vi "Excitation.vi"() -> ()   [LabVIEW 2016]
uses:
  controls/EnumFGVHDT.ctl
  controls/Enum.ctl
  Course Project/support/Message Queue/Message Cluster.ctl
  <vilib>/rvi/errors/niLvFpgaAdjustHostInterfaceError.vi
  <vilib>/rvi/interface/common/niFpgaWaitOnOcc.vi
  <vilib>/RVI Host/nirviSupport.llb/nirviErrorClusterFromErrorCode.vi
  <vilib>/regexp/Match Regular Expression.xnode
  <vilib>/rvi/interface/nirviReadWriteControl/nirviReadWriteControl.xnode
  controls/FPGAVIreferenceTypeDef.ctl
  FPGA Bitfiles/qnmController797_usbRIO_controllerFPGAmu.lvbitx
  <vilib>/rvi/interface/nirviMethod/nirviMethod.xnode
  controls/FPGAVIreferenceTypeDefScanEngine.ctl
  Course Project/support/Message Queue/Message Queue.lvlib
  <vilib>/Analysis/NI_AAL_SigProc.lvlib
  <vilib>/rvi/errors/niLvFpgaMergeErrorWithErrorCode.vi
  NiFpgaLv.dll
  <vilib>/rvi/interface/nirviMethod/StockFPGA_InlinedMethodWaitForSingleIRQ.vi
  Course Project/support/User Event - Stop/User Event - Stop.lvlib
  <vilib>/FPGAPlugInAG/USB-7856R OEM/niLvFpga_AcknowledgeIrq_USB-7856R OEM.vi
  <vilib>/FPGAPlugInAG/USB-7856R OEM/niLvFpga_ConfigureFifo_USB-7856R OEM.vi
  <vilib>/FPGAPlugInAG/USB-7856R OEM/niLvFpga_StartFifo_USB-7856R OEM.vi
  <vilib>/FPGAPlugInAG/USB-7856R OEM/niLvFpga_ReadFifo_USB-7856R OEM.vi
  <vilib>/FPGAPlugInAG/USB-7856R OEM/niLvFpga_StopFifo_USB-7856R OEM.vi
  <vilib>/FPGAPlugInAG/USB-7856R OEM/niLvFpga_WaitOnIrq_USB-7856R OEM.vi
panel:
  in  "ort.bgc.p.waitTicks":u32=4096
  in  "heartBeatSimParams":T1={"curveParams"={"amplitude"=0.2, "peakHeight"=0.05, "cycleLength"=0, "snapIn"=0.001, "adhesion"=0.03, "peakShift"=0, "noiseAmplitude"=0.001, "asymmetry"=0.1}, "cantileverParams"={"samplingRate"=1000000.0, "cantileverFreq"=500000.0, "qFactor"=2.0}} {"cantileverParams"."cantileverFreq" format="%#_6p"; "cantileverParams"."samplingRate" format="%#_6p"}
  in  "lineFitThreshold":dbl=0.02
  in  "intOutMAEnable":bool=TRUE
  in  "Sensitivities":cluster{"Input":dbl, "Output":dbl}={"Input"=0.001506, "Output"=0.00030517578125} {"Output" format="%#_7p"}
  in  "ExcitationTab":enum32{"Page 1"}(tab)
  in  "Excitation enable?":bool caption="Enabling"
  in  "Background":bool
  in  "Signal":u16(ring) items=["Sine Wave", "Triangle Wave", "Square Wave", "Sawtooth Wave", "Heartbeat Signal"]
  in  "Synchronization":T2={"Lower"=0, "Upper"=10000, "Use SyncPoint"=FALSE, "syncPoint"=1000, "Average Band"=4} {"Average Band" items=["1", "2", "4", "16", "32", "64", "128", "256"]}
  out "Graph":dbl[](graph)
  in  "Excitation":T3={"Frequency"=1000.0, "Amplitude"=1e-07, "DC Offset"=0.0, "Cut Off"=40.0, "RaPF"=FALSE, "Shift"=0.0} {"Shift" min=-100.0 max=100.0 format="%_1p%"; "Cut Off" format="%.0p%"; "DC Offset" min=0.0 max=10.0 format="%_3pV"; "Amplitude" min=-10.0 max=10.0 format="%_3pV"; "Frequency" min=0.0 max=100000000.0 format="%.1pHz"}
  in  "Background-":cluster{"Lift Height":dbl, "Average Count":u16}={"Lift Height"=3e-08, "Average Count"=12} {"Average Count" items=["1", "2", "4", "8", "16", "32", "64", "128", "256", "512", "1024", "2048", "4096", "8192", "16384"]; "Lift Height" format="%_3pm"}
  in  "Type":u16(ring) items=["ZPiezo", "Photothermal"]
  in  "Display":u16(ring) items=["Excitation", "Background"]
  in  "Request":enum16{"Never", "End of line", "End of frame"}(ring)
  in  "Correction":bool=TRUE
  # "Excitation"
  # "Background"
  # "Background/Scan"
  # "Maximum search"
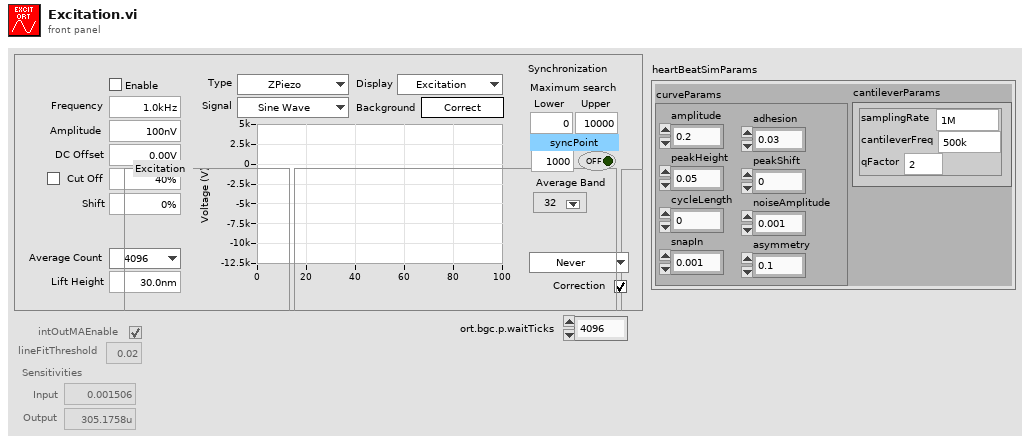
[diagram p1: front panel]
types:
  T1 = cluster{"curveParams":cluster{"amplitude":dbl, "peakHeight":dbl, "cycleLength":u16, "snapIn":dbl, "adhesion":dbl, "peakShift":u16, "noiseAmplitude":dbl, "asymmetry":dbl}, "cantileverParams":cluster{"samplingRate":dbl, "cantileverFreq":dbl, "qFactor":dbl}}
  T2 = cluster{"Lower":u16, "Upper":u16, "Use SyncPoint":bool, "syncPoint":u16, "Average Band":u16}
  T3 = cluster{"Frequency":dbl, "Amplitude":dbl, "DC Offset":dbl, "Cut Off":dbl, "RaPF":bool, "Shift":dbl}
  T4 = typedef "EnumFGVHDT.ctl" = enum16{"Init", "Read", "Write", "Push", "Pop"}
  T5 = typedef "Message Queue.lvlib/All Message Queues.ctl" = cluster{"IU":refnum<queue>}
  T6 = cluster{"Initialization":bool, "Ctrl":refnum<vi>}
  T7 = typedef "Enum.ctl" = enum16{"Init", "Read", "Write"}
  T8 = typedef "Message Queue.lvlib/Message Cluster.ctl" = cluster{"Message":string, "Données de message":variant}
  T9 = cluster{"upperLimit":fxp<+/-,28,4>, "lowerLimit":fxp<+/-,28,4>}
  T10 = enum8{"Enabled", "Disabled", "Disabled and Grayed Out"}
  T11 = cluster{"maxSearchLower":u16, "maxSearchUpper":u16}
  T12 = enum32{"Bad", "Idle", "Run top level", "Running"}
  T13 = cluster{"DC Offset":dbl, "amplitude":dbl, "frequency":dbl, "Signal Type":u16, "cutoff":dbl, "RaPF":bool, "shift":dbl}
  T14 = cluster{"Excitation":cluster{"Frequency":dbl, "Amplitude":dbl, "DC Offset":dbl, "Cut Off":dbl, "RaPF":bool, "Shift":dbl}, "Background":cluster{"Lift Height":dbl, "Average Count":u16}, "Signal":u16}
  T15 = cluster{"DC Offset":dbl, "amplitude":dbl, "frequency":dbl, "Signal Type":u16, "cutoff":dbl, "RaPF":bool}
  T16 = typedef "FPGAVIreferenceTypeDef.ctl" = refnum<k20>
  T17 = cluster{"hdt.int.s.transferSource":u8, "hdt.int.p.useInternalMemStartPos":bool, "hdt.int.p.memStartPos":fxp<+,14,14>, "hdt.int.p.readLength":u16, "hdt.int.p.readFwd":bool, "hdt.int.p.memReadDec":u16, "hdt.int.p.startTransfer":bool}
  T18 = cluster{"ort.p.winSizeP2":u16, "ort.p.syncPoint":u16, "ort.p.useSyncPoint":bool, "ort.p.bypassAvg":bool, "ort.p.searchBounds":cluster{"maxSearchLower":u16, "maxSearchUpper":u16}}
  T19 = typedef "FPGAVIreferenceTypeDefScanEngine.ctl" = refnum<k20>
  T20 = cluster{"calibName":string[], "calibParameters":cluster{"Sensitivity":cluster{"Sens X":dbl, "Sens Y":dbl, "Sens Z":dbl}, "Range":cluster{"Range X":dbl, "Range Y":dbl, "Range Z":dbl}, "HV gain":cluster{"HV gain X":dbl, "HV gain Y":dbl, "HV gain Z":dbl}}[], "calibIndex":i32}
  T21 = cluster{"Sensitivity":cluster{"Sens X":dbl, "Sens Y":dbl, "Sens Z":dbl}, "Range":cluster{"Range X":dbl, "Range Y":dbl, "Range Z":dbl}, "HV gain":cluster{"HV gain X":dbl, "HV gain Y":dbl, "HV gain Z":dbl}}[]
  T22 = cluster{"Sensitivity":cluster{"Sens X":dbl, "Sens Y":dbl, "Sens Z":dbl}, "Range":cluster{"Range X":dbl, "Range Y":dbl, "Range Z":dbl}, "HV gain":cluster{"HV gain X":dbl, "HV gain Y":dbl, "HV gain Z":dbl}}
  T23 = cluster{"liftHeight":fxp<+/-,15,4>, "disengagePos":fxp<+/-,22,1>}
  T24 = cluster{"maxSearchLower":u16, "maxSearchUpper":u16, "useSyncPoint":bool, "syncPoint":u16, "syncAverageBand":u16}
  T25 = cluster{"inputSensitivity":dbl, "outputSensitivity":dbl}
  T26 = cluster{"intOutMAEnable":bool, "bgcAverageCount":u16, "waveSize":u32, "resetBGC":bool, "liftHeight":fxp<+/-,15,4>}
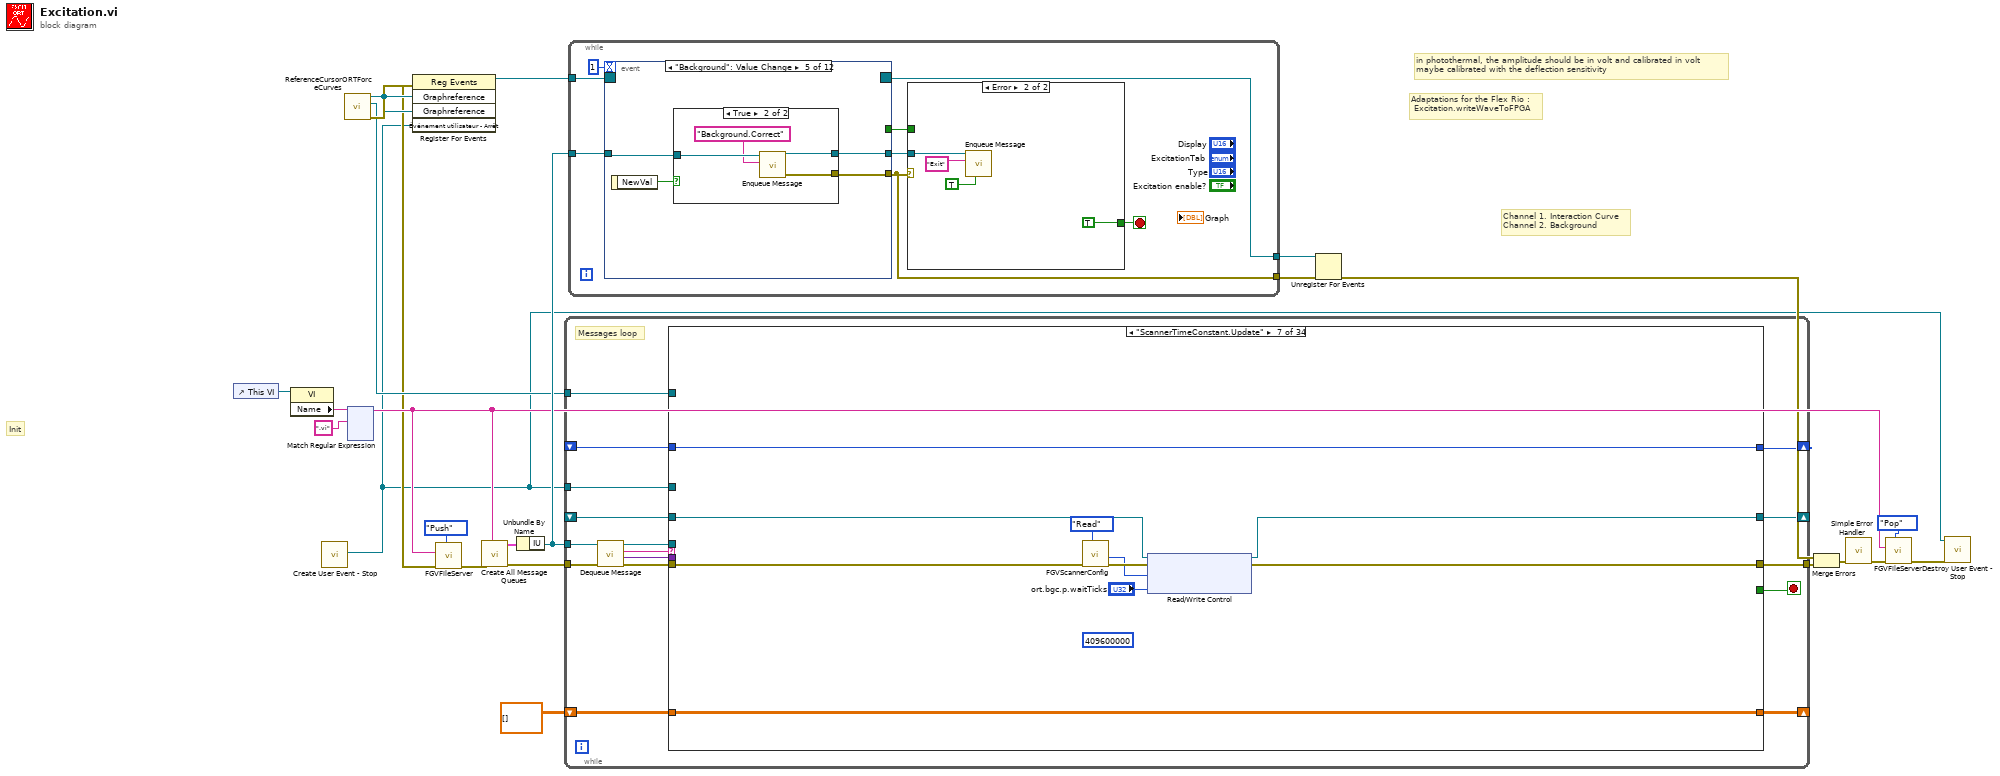
[diagram p0: block diagram]
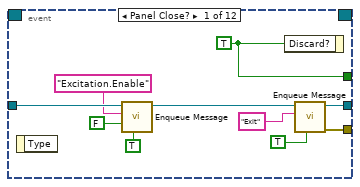
[diagram p3: hidden frame]
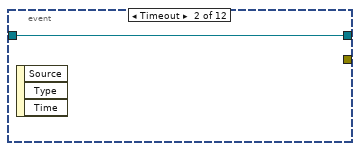
[diagram p4: hidden frame]
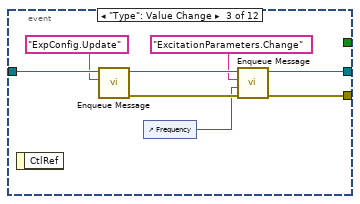
[diagram p5: hidden frame]
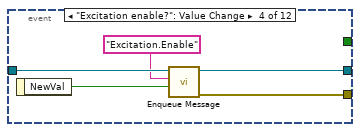
[diagram p6: hidden frame]
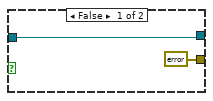
[diagram p7: hidden frame]
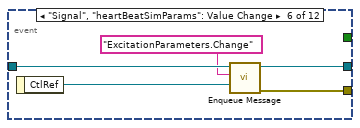
[diagram p8: hidden frame]
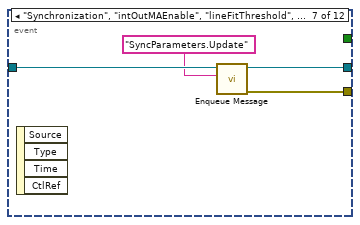
[diagram p9: hidden frame]
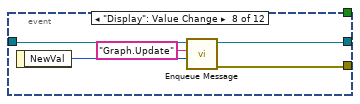
[diagram p10: hidden frame]
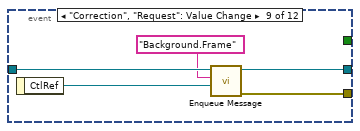
[diagram p11: hidden frame]
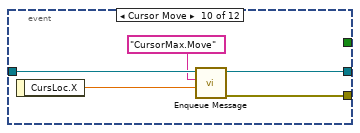
[diagram p12: hidden frame]
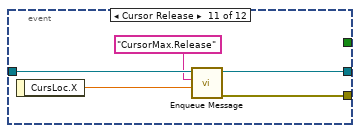
[diagram p13: hidden frame]
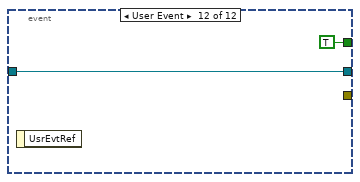
[diagram p14: hidden frame]
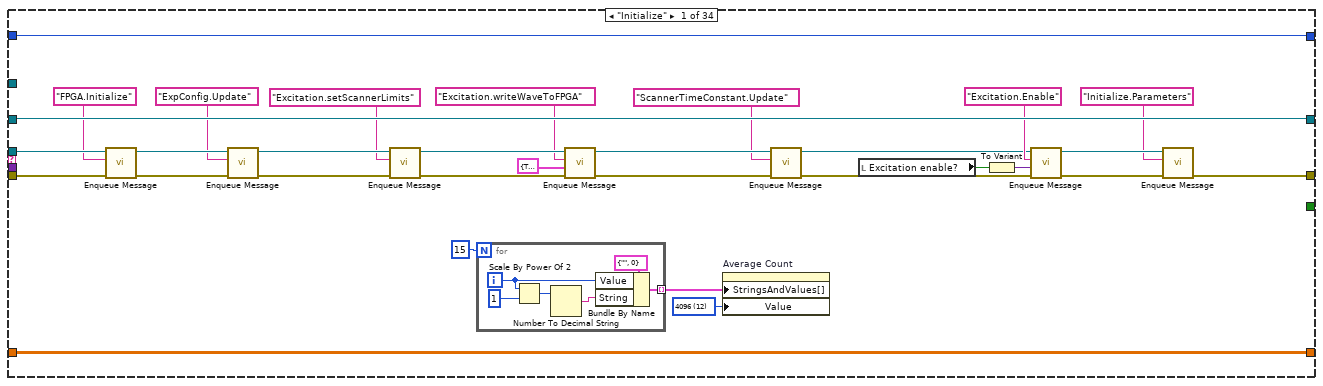
[diagram p15: hidden frame]
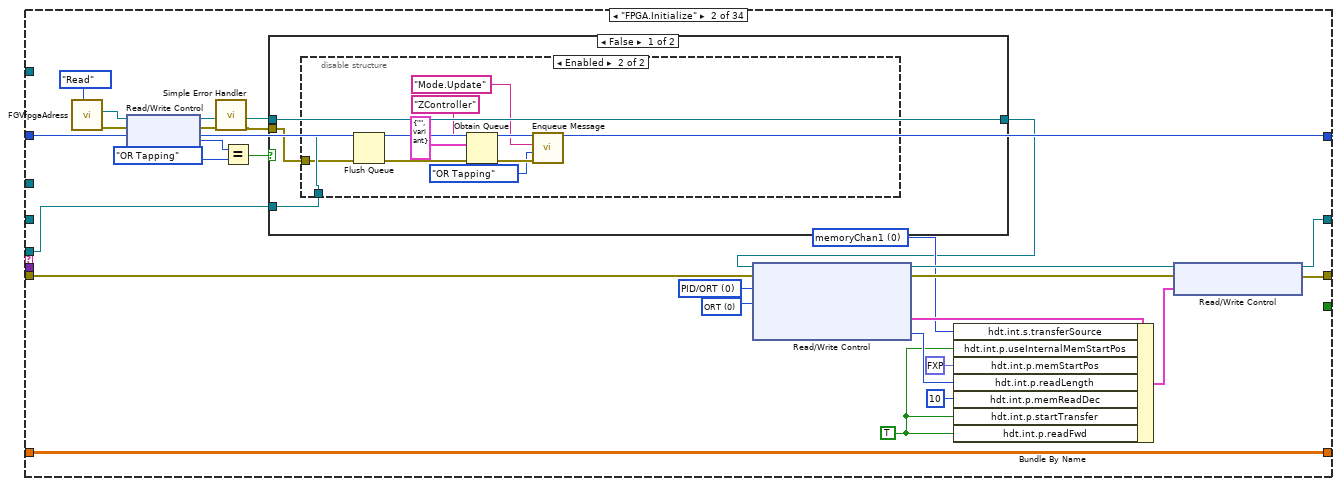
[diagram p16: hidden frame]
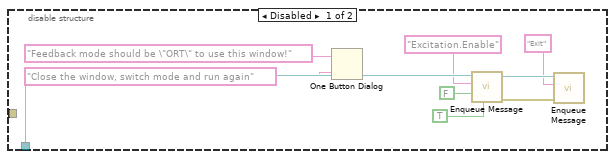
[diagram p17: hidden frame]
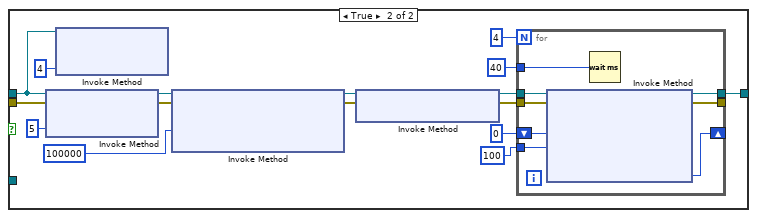
[diagram p18: hidden frame]
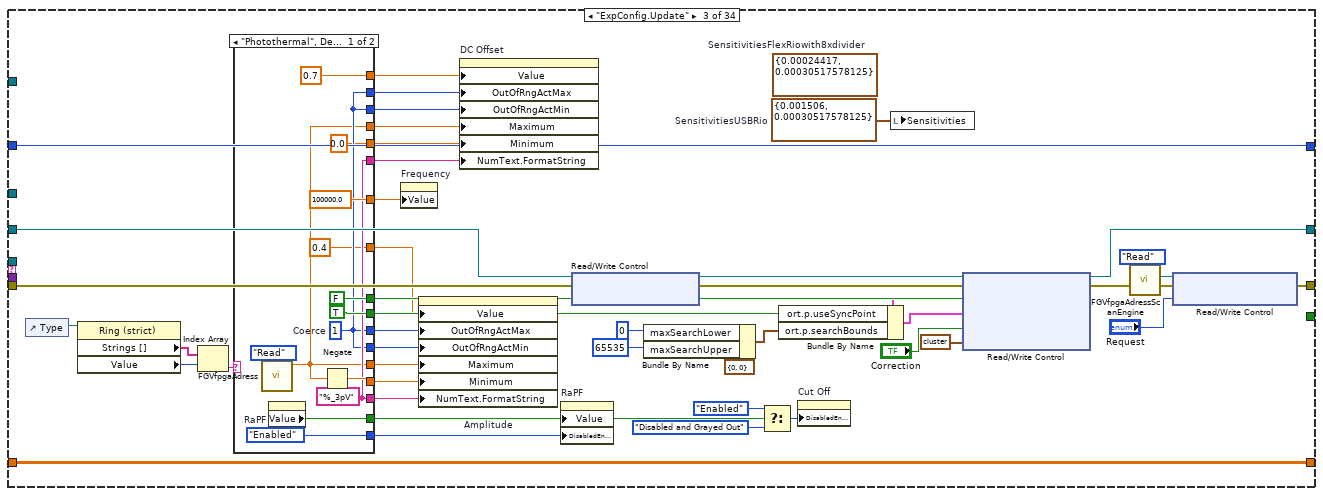
[diagram p19: hidden frame]
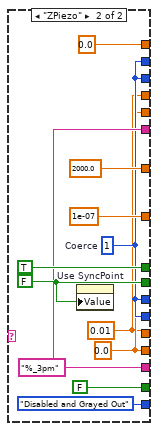
[diagram p20: hidden frame]
diagram:
  # "Adaptations for the Flex Rio : \n Excitation.writeWaveToFPGA"
  # "Channel 1. Interaction Curve\nChannel 2. Background"
  # "Init"
  # "in photothermal, the amplitude should be in volt and calibrated in volt\nmaybe calibrated with the deflection sensitivity"
  n1 = control-ref of="This VI"() -> (w13:refnum<vi>)
  n2 = property class="VI"(reference=w13) -> ("Name"=w12:string)  [unwired: 1 in, 2 out]
  n3 = call "Create User Event - Stop.vi"() -> ("Événement utilisateur - Arrêt"=w1:refnum<user-event>)  [unwired: 9 in, 2 out]
  n4 = call "ReferenceCursorORTForceCurves.vi"() -> ("error out"=w24:errorcluster, "vi reference"=w15:refnum<vi>, "Graphreference"=w14:refnum<vi>)  [unwired: 9 in]
  n5 = xnode "Match Regular Expression"("input string"=w12, "regular expression"=".vi") -> ("before match"=w5:string)  [unwired: 4 in, 4 out]
  n6 = register-events(error in=w24, w14, w14, w1) -> (reference out=w17:refnum<event-registration>, error out=w3:errorcluster)  [unwired: 1 in]
  n7 = call "FGVFileServer.vi"("Enum"=EnumFGVHDT."Push", "error in"=w3, "New VI"=w5) -> ("error out"=w9:errorcluster)  [unwired: 7 in, 1 out]
  n8 = call "Create All Message Queues.vi"("QueueName"=w5, "ErrorIn"=w9) -> ("ErrorOut"=w19:errorcluster, "MessageQueueOut"=w20:T5)  [unwired: 8 in]
  n9 = Unbundle By Name(w20) -> ("IU"=w22:refnum<queue>)
  n10 = while {
    tunnel: w22 -> [w35]
    shift-right: [w34] -> _
    shift-left: _ -> [w33]
    shift-right: [w32] -> _
    shift-left: _ -> [w31]
    shift-right: [w29] -> _
    shift-left: dbl[][] [] -> [w30]
    tunnel: w19 -> [w39]
    tunnel: [w28] -> w21
    tunnel: w15 -> [w26]
    tunnel: w1 -> [w25]
    stop <- w40 stop-if-true
    # "Messages loop"
    n11 = call "Dequeue Message.vi"("entrée d'erreur (pas d'erreur)"=w39, "File d'attente de messages"=w35) -> ("sortie d'erreur"=w38:errorcluster, "Données de message"=w37:variant, "Message"=w27:string, "File d'attente de message dup."=w36:refnum<queue>)  [unwired: 6 in]
    n12 = case shown="\"ScannerTimeConstant.Update\"" w27 {
      selector: w27 -> [_ _ _ _ _ _ _ _ _ _ _ _ _ _ _ _ _ _ _ _ _ _ _ _ _ _ _ _ _ _ _ _ w989 _]
      tunnel: w36 -> [w66 w78 _ w235 w283 _ _ _ _ w345 w422 _ _ w544 _ w626 _ _ _ _ _ _ _ _ _ _ _ _ w929 _ _ _ _ _]
      tunnel: w38 -> [w67 w102 w178 w234 w281 w290 w301 w310 w318 w339 w387 w482 w532 w536 w591 w615 w689 w731 w757 w805 w808 w835 w877 w891 w896 w905 w917 w921 w924 w949 w976 w982 _ w1007]
      tunnel: [w60 w89 w154 w233 w278 w292 w302 w310 w314 w344 w384 w473 w532 w539 w586 w618 w698 w721 w757 w790 w807 w872 w886 w891 w895 w905 w909 w921 w923 w946 w967 w981 w987 w1008] -> w28
      tunnel: [_ _ _ _ TRUE _ _ _ _ _ _ _ _ _ _ _ _ _ _ _ _ _ _ _ _ _ _ _ _ _ _ _ _ _] -> w40
      tunnel: w37 -> [_ _ _ _ _ w291 _ _ w320 w337 w414 _ _ _ _ _ _ w730 _ _ _ _ _ _ _ _ _ _ _ w948 w975 _ _ _]
      tunnel: [w69 w90 w152 w219 w261 w295 w299 w308 w316 w327 w444 w478 w531 w533 w562 w619 w688 w722 w755 w802 w815 w866 w884 w890 w900 w904 w907 w919 w928 w943 w968 w978 w984 w1009] -> w34
      tunnel: w33 -> [w69 _ w179 w231 w263 w296 w300 w308 w319 w328 w445 w479 w531 w534 w610 w621 w688 w723 w755 w806 w815 w834 w878 w890 w900 w904 w908 w919 w928 w943 w970 w978 w984 w1009]
      tunnel: [w64 w104 w192 w229 w280 w294 w306 w309 w315 w343 w423 w505 w530 w542 w584 w616 w696 w720 w756 w775 w811 w845 w879 w889 w901 w903 w911 w918 w927 w944 w966 w979 w983 w993] -> w32
      tunnel: w31 -> [w64 w104 w192 w229 w280 w294 w306 w309 w315 w343 _ w505 w530 w542 w584 w616 w696 w720 w756 w775 w811 w845 w879 w889 w901 w903 w911 w918 w927 w944 w966 w979 w983 w993]
      tunnel: [w63 w103 w193 w232 w279 w293 w305 w307 w313 w341 w424 w475 w529 w541 w581 w620 w693 w719 w754 w795 w810 w862 w882 w888 w899 w902 w906 w920 w926 w945 w965 w980 w985 w994] -> w29
      tunnel: w30 -> [w63 w103 w193 w232 w279 w293 w305 w307 w313 w341 _ w475 w529 w541 w582 w620 w694 w719 w754 w795 w810 w846 w880 w888 w899 w902 w906 w920 w926 w945 w965 w980 w985 w994]
      tunnel: w26 -> [_ _ _ _ w277 _ _ _ _ _ _ _ _ _ _ _ _ _ _ _ _ _ _ _ _ _ _ _ _ _ _ _ _ _]
      tunnel: w25 -> [_ _ _ _ w258 _ _ _ _ _ _ _ _ _ _ _ _ _ _ _ _ _ _ _ _ _ _ _ _ _ _ _ _ _]
      frame "Initialize" {
        w53 = u16 12 items=["1", "2", "4", "8", "16", "32", "64", "128", "256", "512", "1024", "2048", "4096", "8192", "16384"] ("bgcAverageCount")
        n13 = call "Enqueue Message.vi"("error in"=w67, "Message"="FPGA.Initialize", "Queue"=w66) -> ("error out"=w61:errorcluster, "Queue dup."=w62:refnum<queue>)  [unwired: 7 in]
        n14 = call "Enqueue Message.vi"("error in"=w61, "Message"="ExpConfig.Update", "Queue"=w62) -> ("error out"=w48:errorcluster, "Queue dup."=w49:refnum<queue>)  [unwired: 7 in]
        n15 = call "Enqueue Message.vi"("error in"=w48, "Message"="Excitation.setScannerLimits", "Queue"=w49) -> ("error out"=w47:errorcluster, "Queue dup."=w70:refnum<queue>)  [unwired: 7 in]
        n16 = for {
          N: 15 -> [_]
          tunnel: [w72] -> w54 mode=indexing
          i -> [w75]
          n17 = Scale By Power Of 2(n=w75, x=i16 1 ("n")) -> (x*2^n=w74:i16)
          n18 = Number To Decimal String(number=w74) -> (decimal integer string=w73:string)  [unwired: 1 in]
          n19 = Bundle By Name(cluster=cluster{"String":string, "Value":u16} {"String"="", "Value"=0} ("Cluster"), "Value"=w75, "String"=w73) -> (w72:cluster{"String":string, "Value":u16})
        }
        n20 = call "Enqueue Message.vi"("error in"=w47, "Data"=T6 {"Initialization"=TRUE, "Ctrl"=refnum}, "Message"="Excitation.writeWaveToFPGA", "Queue"=w70) -> ("error out"=w43:errorcluster, "Queue dup."=w71:refnum<queue>)  [unwired: 6 in]
        n21 = property on="Average Count" class="Ring (strict)"("StringsAndValues[]"=w54, "Value"=w53) -> ()  [unwired: 2 in, 2 out]
        n22 = call "Enqueue Message.vi"("error in"=w43, "Message"="ScannerTimeConstant.Update", "Queue"=w71) -> ("error out"=w42:errorcluster, "Queue dup."=w41:refnum<queue>)  [unwired: 7 in]
        n23 = local read "Excitation enable?"() -> (w56:bool)
        n24 = To Variant(anything=w56) -> (Variant=w45:variant)
        n25 = call "Enqueue Message.vi"("error in"=w42, "Data"=w45, "Message"="Excitation.Enable", "Queue"=w41) -> ("error out"=w51:errorcluster, "Queue dup."=w68:refnum<queue>)  [unwired: 6 in]
        n26 = call "Enqueue Message.vi"("error in"=w51, "Message"="Initialize.Parameters", "Queue"=w68) -> ("error out"=w60:errorcluster)  [unwired: 7 in, 1 out]
      }
      frame "FPGA.Initialize" {
        w101 = u8 0 items=["ORT", "SICM"] ("hdt.int.p.memWriteSource")
        w100 = u8 0 items=["PID/ORT", "SICM"] ("hdt.mainOutStreamSelect")
        w91 = TRUE ("hdt.int.p.startTransfer")
        w94 = u8 0 items=["memoryChan1", "memoryChan2", "processVarFixedNoPts", "processVarStream"] ("hdt.int.s.transferSource")
        n27 = call "FGVfpgaAdress.vi"("Enum"=Enum."Read") -> ("error out"=w81:errorcluster, "FPGA VI Reference Out"=w87:T16)  [unwired: 5 in, 4 out]
        n28 = xnode "Read/Write Control"("FPGA VI Reference In"=w87, "error in"=w81) -> ("FPGA VI Reference Out"=w86:T16, "error out"=w82:errorcluster, "fb.i.source"=w85:u8)
        n29 = call <vilib>:"Simple Error Handler.vi"("error in (no error)"=w82) -> ("error out"=w80:errorcluster)  [unwired: 4 in, 4 out]
        n30 = Equal?(x=w85, y=enum16{"Contact", "OR Tapping", "Aux"}."OR Tapping" ("Mode")) -> (x = y?=w83:bool)
        n31 = case shown="False" w83 {
          tunnel: [w106 w129] -> w79
          tunnel: w86 -> [w106 w127]
          tunnel: w80 -> [w105 w131]
          tunnel: w78 -> [w107 _]
          frame False {
            n32 = disable-structure shown="Enabled" {
              disable-tunnel: w107 -> [w115 w119]
              disable-tunnel: w105 -> [_ w118]
              frame Disabled {
                n33 = One Button Dialog(message="Feedback mode should be \"ORT\" to use this window!" ("Message"), button name ("OK")="Close the window, switch mode and run again") -> ()  [unwired: 1 out]
                n34 = call "Enqueue Message.vi"("Prioritary message"=TRUE, "Data"=FALSE, "Message"="Excitation.Enable", "Queue"=w115) -> ("error out"=w108:errorcluster, "Queue dup."=w116:refnum<queue>)  [unwired: 6 in]
                n35 = call "Enqueue Message.vi"("error in"=w108, "Message"="Exit" ("QueueName"), "Queue"=w116) -> ()  [unwired: 7 in, 2 out]
              }
              frame Enabled {
                n36 = Flush Queue(queue=w119, error in (no error)=w118) -> (error out=w117:errorcluster)  [unwired: 2 out]
                n37 = Obtain Queue(name (unnamed)="ZController" ("QueueName"), element data type=T8 {"Message"="", "Données de message"=variant} ("Cluster Message"), error in (no error)=w117) -> (queue out=w124:refnum<queue>, error out=w125:errorcluster)  [unwired: 2 in, 1 out]
                n38 = call "Enqueue Message.vi"("error in"=w125, "Data"=enum16{"Contact", "OR Tapping", "Aux"}."OR Tapping" ("Mode"), "Message"="Mode.Update", "Queue"=w124) -> ()  [unwired: 6 in, 2 out]
              }
            }
          }
          frame True {
            n39 = xnode "Invoke Method"("FPGA VI Reference In"=w127, "error in"=w131, "IRQ Number(s)"=5) -> ("FPGA VI Reference Out"=w133:T16, "error out"=w134:errorcluster)
            n40 = xnode "Invoke Method"("FPGA VI Reference In"=w127, "IRQ Number(s)"=4) -> ()  [unwired: 1 in, 2 out]
            n41 = xnode "Invoke Method"("FPGA VI Reference In"=w133, "error in"=w134, "Requested Depth"=u32 100000) -> ("FPGA VI Reference Out"=w137:T16, "error out"=w135:errorcluster)  [unwired: 1 out]
            n42 = xnode "Invoke Method"("FPGA VI Reference In"=w137, "error in"=w135) -> ("FPGA VI Reference Out"=w138:T16, "error out"=w141:errorcluster)
            n43 = for {
              N: 4 -> [_]
              shift-right: [w144] -> _
              shift-left: u32 0 ("Elements Remaining") -> [w145]
              tunnel: 100 ("Timeout (ms)") -> [w143]
              tunnel: w138 -> [w149]
              tunnel: [w147] -> w129
              tunnel: w141 -> [w148]
              tunnel: [w146] -> _
              tunnel: u32 40 ("milliseconds to wait") -> [w142]
              n44 = xnode "Invoke Method"("FPGA VI Reference In"=w149, "error in"=w148, "Number of Elements"=w145, "Timeout (ms)"=w143) -> ("FPGA VI Reference Out"=w147:T16, "error out"=w146:errorcluster, "Elements Remaining"=w144:u32)  [unwired: 1 out]
              n45 = Wait (ms)(milliseconds to wait=w142) -> ()  [unwired: 1 out]
            }
          }
        }
        n46 = xnode "Read/Write Control"("FPGA VI Reference In"=w79, "error in"=w102, "hdt.mainOutStreamSelect"=w100, "hdt.int.p.memWriteSource"=w101) -> ("FPGA VI Reference Out"=w97:T16, "error out"=w98:errorcluster, "hdt.int.p.readParams"=w95:T17, "ort.p.waveSize"=w96:u16)
        n47 = Bundle By Name(cluster=w95, "hdt.int.s.transferSource"=w94, "hdt.int.p.useInternalMemStartPos"=w91, "hdt.int.p.memStartPos"=fxp<+,14,14> 0.0, "hdt.int.p.readLength"=w96, "hdt.int.p.memReadDec"=u16 10, "hdt.int.p.startTransfer"=w91, "hdt.int.p.readFwd"=w91) -> (w99:T17)
        n48 = xnode "Read/Write Control"("FPGA VI Reference In"=w97, "error in"=w98, "hdt.int.p.readParams"=w99) -> ("FPGA VI Reference Out"=w90:T16, "error out"=w89:errorcluster)
      }
      frame "ExpConfig.Update" {
        w150 = cluster{"Input":dbl, "Output":dbl} {"Input"=0.001506, "Output"=0.00030517578125}  # SensitivitiesUSBRio
        (unwired) cluster{"Input":dbl, "Output":dbl} {"Input"=0.00024417, "Output"=0.00030517578125}  # SensitivitiesFlexRiowith8xdivider
        n49 = control-ref of="Type"() -> (w191:refnum<vi>)
        n50 = property class="Ring (strict)"(reference=w191) -> ("Strings []"=w190:string[], "Value"=w189:u16)  [unwired: 1 in, 2 out]
        n51 = Index Array(array=w190, index=w189) -> (element=w188:string)
        n52 = case shown="\"Photothermal\", Default" w188 {
          tunnel: [FALSE ("piezoMode") TRUE ("piezoMode")] -> w194
          tunnel: [TRUE ("piezoMode") w217] -> w182
          tunnel: [w205 FALSE ("Value")] -> w175
          tunnel: [T10."Enabled" ("Disabled") T10."Disabled and Grayed Out" ("Disabled")] -> w171
          tunnel: [w200 w212] -> w170
          tunnel: [w202 w210] -> w169
          tunnel: [w195 w209] -> w168
          tunnel: [w199 w211] -> w167
          tunnel: [w199 w211] -> w166
          tunnel: [0.4 1e-07] -> w165
          tunnel: [100000.0 2000.0] -> w164
          tunnel: [w200 w212] -> w163
          tunnel: [w199 w211] -> w162
          tunnel: [w199 w211] -> w161
          tunnel: [w195 w209] -> w160
          tunnel: [0.0 ("voltageRange(+/-)Out") w210] -> w159
          tunnel: [0.7 0.0] -> w158
          frame "Photothermal", Default {
            w199 = u8 1  # Coerce
            w200 = "%_3pV" ("Numeric Text.Format String")
            n53 = call "FGVfpgaAdress.vi"("Enum"=Enum."Read") -> ("voltageRange(+/-)Out"=w195:dbl)  [unwired: 5 in, 5 out]
            n54 = property on="RaPF" class="Bool (strict)"() -> ("Value"=w205:bool)  [unwired: 2 in, 2 out]
            n55 = Negate(x=w195) -> (-x=w202:dbl)
          }
          frame "ZPiezo" {
            w209 = 0.01 ("voltageRange(+/-)Out")
            w211 = u8 1  # Coerce
            w210 = 0.0
            w212 = "%_3pm" ("Numeric Text.Format String")
            w217 = FALSE ("piezoMode")
            n56 = property on="Use SyncPoint" class="Bool (strict)"("Value"=w217) -> ()  [unwired: 2 in, 2 out]
          }
        }
        n57 = property on="Frequency" class="DigNum (strict)"("Value"=w164) -> ()  [unwired: 2 in, 2 out]
        n58 = property on="Amplitude" class="DigNum (strict)"("Value"=w165, "OutOfRngActMax"=w167, "OutOfRngActMin"=w166, "Maximum"=w168, "Minimum"=w169, "NumText.FormatString"=w170) -> ()  [unwired: 2 in, 2 out]
        n59 = property on="DC Offset" class="DigNum (strict)"("Value"=w158, "OutOfRngActMax"=w161, "OutOfRngActMin"=w162, "Maximum"=w160, "Minimum"=w159, "NumText.FormatString"=w163) -> ()  [unwired: 2 in, 2 out]
        n60 = property on="RaPF" class="Bool (strict)"("Value"=w175, "DisabledEnum"=w171) -> ()  [unwired: 2 in, 2 out]
        n61 = xnode "Read/Write Control"("FPGA VI Reference In"=w179, "error in"=w178) -> ("FPGA VI Reference Out"=w180:T16, "error out"=w177:errorcluster, "ort.p.methodParams"=w184:T18)
        n62 = Bundle By Name(cluster=T11 {"maxSearchLower"=0, "maxSearchUpper"=0} ("maxSearchBounds"), "maxSearchLower"=u16 0, "maxSearchUpper"=u16 65535) -> (w181:T11)
        n63 = Select(t=T10."Enabled" ("Disabled"), s=w175, f=T10."Disabled and Grayed Out" ("Disabled")) -> (s? t:f=w172:T10)
        n64 = Bundle By Name(cluster=w184, "ort.p.useSyncPoint"=w182, "ort.p.searchBounds"=w181) -> (w183:T18)
        n65 = property on="Cut Off" class="DigNum (strict)"("DisabledEnum"=w172) -> ()  [unwired: 2 in, 2 out]
        n66 = local write "Sensitivities"(w150) -> ()
        n67 = xnode "Read/Write Control"("FPGA VI Reference In"=w180, "error in"=w177, "ort.o.piezoMode"=w194, "ort.p.methodParams"=w183, "itc.p.allowBGC"="Correction", "fb.p.limits"=T9 {"upperLimit"=1.0, "lowerLimit"=-1.0}) -> ("FPGA VI Reference Out"=w152:T16, "error out"=w153:errorcluster)
        n68 = call "FGVfpgaAdressScanEngine.vi"("Enum"=Enum."Read") -> ("FPGA.SEout"=w156:T19)  [unwired: 6 in, 4 out]
        n69 = xnode "Read/Write Control"("FPGA VI Reference In"=w156, "error in"=w153, "ort.bgc.requestType"="Request") -> ("error out"=w154:errorcluster)  [unwired: 1 out]
      }
      frame "Initialize.Parameters" {
        # "When initializing, assume the sync point is at about the middle of the wave"
        n70 = xnode "Read/Write Control"("FPGA VI Reference In"=w231, "error in"=w234) -> ("FPGA VI Reference Out"=w219:T16, "error out"=w224:errorcluster, "fb.p.enable"=w230:bool)
        n71 = local read "lineFitThreshold"() -> (w227:dbl)
        n72 = local read "Synchronization"() -> (w226:T2)
        n73 = local read "Sensitivities"() -> (w225:cluster{"Input":dbl, "Output":dbl})
        n74 = call "Enqueue Message.vi"("error in"=w224, "Message"="SyncParameters.Reset", "Queue"=w235) -> ("error out"=w222:errorcluster, "Queue dup."=w221:refnum<queue>)  [unwired: 7 in]
        n75 = call "Enqueue Message.vi"("error in"=w222, "Message"="Interaction.updateParameters", "Queue"=w221) -> ("error out"=w237:errorcluster, "Queue dup."=w236:refnum<queue>)  [unwired: 7 in]
        n76 = call "FGVExcitationParameters.vi"("Enum"=Enum."Write", "error in"=w237, "lineFitThreshold In"=w227, "syncParameters In"=w226, "Sensitivities In"=w225) -> ("error out"=w238:errorcluster)  [unwired: 2 in, 4 out]
        n77 = case shown="True" w230 {
          tunnel: [w239 w247] -> w233
          tunnel: w236 -> [_ w246]
          tunnel: w238 -> [w239 w241]
          tunnel: w229 -> [_ w240]
          frame False {
          }
          frame True {
            n78 = control-ref of="Type"() -> (w245:refnum<vi>)
            n79 = property class="Ring (strict)"(reference=w245, error in=w241) -> (error out=w248:errorcluster, "Strings []"=w244:string[], "Value"=w243:u16)  [unwired: 1 out]
            n80 = Index Array(array=w244, index=w243) -> (element=w242:string)
            n81 = case shown="\"ZPiezo\"" w242 {
              tunnel: [w253 w255] -> w247
              tunnel: w246 -> [_ w257]
              tunnel: w248 -> [w253 w254]
              tunnel: w240 -> [w249 _]
              frame "ZPiezo" {
                n82 = local read "Synchronization"() -> (w252:T2)
                n83 = Bundle By Name(cluster=w252, "Upper"=w249, "Use SyncPoint"=TRUE ("useSyncPoint")) -> (w250:T2)
                n84 = local write "Synchronization"(w250) -> ()
              }
              frame "Photothermal", Default {
                n85 = call "Enqueue Message.vi"("error in"=w254, "Message"="SyncParameters.Update", "Queue"=w257) -> ("error out"=w255:errorcluster)  [unwired: 7 in, 1 out]
              }
            }
          }
        }
      }
      frame "Exit" {
        w265 = u8 2 items=["memoryChan1", "memoryChan2", "processVarFixedNoPts", "processVarStream"] ("hdt.int.s.transferSource")
        n86 = property class="VI"(reference=w277) -> (reference out=w276:refnum<vi>, "Exec.State"=w274:T12)  [unwired: 1 in, 1 out]
        n87 = Release Queue(queue=w283, error in (no error)=w281) -> (error out=w264:errorcluster)  [unwired: 1 in, 2 out]
        n88 = Equal?(x=T12."Running" ("Execution:State"), y=w274) -> (x = y?=w271:bool)
        n89 = Equal?(x=w274, y=T12."Run top level" ("Execution:State")) -> (x = y?=w272:bool)
        n90 = Or(x=w271, y=w272) -> (x .or. y?=w270:bool)
        n91 = case shown="True" w270 {
          tunnel: w276 -> [_ w285]
          frame False {
          }
          frame True {
            n92 = invoke class="VI" method="Abort VI"(reference=w285) -> (reference out=w284:refnum<vi>)  [unwired: 2 in, 2 out]
            n93 = Close Reference(reference=w284) -> ()  [unwired: 1 in, 1 out]
          }
        }
        n94 = call "Fire User Event - Stop.vi"("Événement utilisateur - Arrêt"=w258) -> ()  [unwired: 10 in, 1 out]
        n95 = xnode "Read/Write Control"("FPGA VI Reference In"=w263, "error in"=w264) -> ("FPGA VI Reference Out"=w267:T16, "error out"=w268:errorcluster, "hdt.int.p.readParams"=w266:T17)
        n96 = Bundle By Name(cluster=w266, "hdt.int.s.transferSource"=w265) -> (w269:T17)
        n97 = xnode "Read/Write Control"("FPGA VI Reference In"=w267, "error in"=w268, "hdt.int.p.readParams"=w269) -> ("FPGA VI Reference Out"=w262:T16, "error out"=w260:errorcluster)
        n98 = xnode "Invoke Method"("FPGA VI Reference In"=w262, "error in"=w260) -> ("FPGA VI Reference Out"=w261:T16, "error out"=w259:errorcluster)
        n99 = Merge Errors(w259) -> (w278:errorcluster)
      }
      frame "Feedback.Disable" {
        n100 = Variant To Data(error in=w290, type=TRUE, Variant=w291) -> (data=w287:bool, error out=w289:errorcluster)
        n101 = Not(x=w287) -> (.not. x?=w286:bool)
        n102 = xnode "Read/Write Control"("FPGA VI Reference In"=w296, "error in"=w289, "fb.p.enable"=w286) -> ("FPGA VI Reference Out"=w295:T16, "error out"=w292:errorcluster)
      }
      frame "ScannerTimeConstant.Update" {
        (unwired) u32 409600000 ("ort.bgc.p.waitTicks")
        n103 = call "FGVScannerConfig.vi"("Enum"=Enum."Read", "error in"=w301) -> ("error out"=w303:errorcluster, "scannerTimeConstantOut"=w298:u16)  [unwired: 7 in, 1 out]
        n104 = xnode "Read/Write Control"("FPGA VI Reference In"=w300, "error in"=w303, "ort.bgc.p.scannerTc"=w298, "ort.bgc.p.waitTicks"="ort.bgc.p.waitTicks") -> ("FPGA VI Reference Out"=w299:T16, "error out"=w302:errorcluster)
      }
      frame "--------- Excitation ----------" {
      }
      frame "Excitation.Enable" {
        n105 = Variant To Data(error in=w318, type=TRUE, Variant=w320) -> (data=w311:bool, error out=w321:errorcluster)
        n106 = property on="Excitation enable?" class="Bool (strict)"(error in=w321, "Value"=w311) -> (error out=w322:errorcluster)  [unwired: 1 in, 1 out]
        n107 = Not(x=w311) -> (.not. x?=w312:bool)
        n108 = xnode "Read/Write Control"("FPGA VI Reference In"=w319, "error in"=w322, "aio.o.disableExc"=w312) -> ("FPGA VI Reference Out"=w316:T16, "error out"=w314:errorcluster)
      }
      frame "ExcitationParameters.Change" {
        # "If the Excitation is on, we should turn it off before changing parameters"
        n109 = local read "Excitation enable?"() -> (w340:bool)
        n110 = Variant To Data(error in=w339, type=refnum<vi> refnum ("CtlRef"), Variant=w337) -> (data=w332:refnum<vi>, error out=w338:errorcluster)
        n111 = case shown="True" w340 {
          tunnel: w345 -> [w375 w381]
          tunnel: [w375 w380] -> w347
          tunnel: [w374 w378] -> w329
          tunnel: w338 -> [w374 w377]
          frame False {
          }
          frame True {
            n112 = call "Enqueue Message.vi"("error in"=w377, "Data"=FALSE ("Excitation enable?"), "Message"="Excitation.Enable", "Queue"=w381) -> ("error out"=w378:errorcluster, "Queue dup."=w380:refnum<queue>)  [unwired: 6 in]
          }
        }
        n113 = xnode "Read/Write Control"("FPGA VI Reference In"=w328, "error in"=w329) -> ("FPGA VI Reference Out"=w327:T16, "error out"=w330:errorcluster, "fb.p.enable"=w326:bool)
        n114 = case shown="True" w326 {
          tunnel: [w360 w367] -> w325
          tunnel: w347 -> [w360 w366]
          tunnel: [w361 w365] -> w324
          tunnel: w330 -> [w361 w362]
          frame False {
          }
          frame True {
            n115 = call "Enqueue Message.vi"("error in"=w362, "Data"=TRUE, "Message"="Feedback.Disable", "Queue"=w366) -> ("error out"=w365:errorcluster, "Queue dup."=w367:refnum<queue>)  [unwired: 6 in]
          }
        }
        n116 = call "Enqueue Message.vi"("error in"=w324, "Message"="Excitation.setScannerLimits", "Queue"=w325) -> ("error out"=w350:errorcluster, "Queue dup."=w351:refnum<queue>)  [unwired: 7 in]
        n117 = Bundle By Name(cluster=T6 {"Initialization"=TRUE, "Ctrl"=refnum}, "Initialization"=FALSE, "Ctrl"=w332) -> (w335:T6)
        n118 = call "Enqueue Message.vi"("error in"=w350, "Data"=w335, "Message"="Excitation.writeWaveToFPGA", "Queue"=w351) -> ("error out"=w346:errorcluster, "Queue dup."=w348:refnum<queue>)  [unwired: 6 in]
        n119 = case shown="True" w326 {
          tunnel: [w353 w359] -> w349
          tunnel: w348 -> [w353 w358]
          tunnel: w346 -> [w352 w357]
          tunnel: [w352 w355] -> w331
          frame False {
          }
          frame True {
            n120 = call "Enqueue Message.vi"("error in"=w357, "Data"=FALSE, "Message"="Feedback.Disable", "Queue"=w358) -> ("error out"=w355:errorcluster, "Queue dup."=w359:refnum<queue>)  [unwired: 6 in]
          }
        }
        n121 = case shown="True" w340 {
          tunnel: w349 -> [_ w373]
          tunnel: w331 -> [w368 w371]
          tunnel: [w368 w370] -> w344
          frame False {
          }
          frame True {
            n122 = call "Enqueue Message.vi"("error in"=w371, "Data"=TRUE ("Excitation enable?"), "Message"="Excitation.Enable", "Queue"=w373) -> ("error out"=w370:errorcluster)  [unwired: 6 in, 1 out]
          }
        }
      }
      frame "Excitation.writeWaveToFPGA" {
        w398 = u16 1 items=["ZPiezo", "Photothermal"] ("Type")
        w393 = 1.0 ("t")
        w407 = 100.0  # Percent
        # "If Piezo, a factor of 10V (Amplifier) should be divided"
        # "Display \"real\" frequency"
        # "When excitation is changed,\nmost likely the background is no longer valid. Set zero to reflect this assumption."
        # "Background"
        # "Excitation"
        n123 = Variant To Data(type=T6 {"Initialization"=TRUE, "Ctrl"=refnum}, Variant=w414) -> (data=w418:T6, error out=w417:errorcluster)  [unwired: 1 in]
        n124 = property on="Excitation enable?" class="Bool (strict)"(error in=w387, "BoolText.Text"="Loading..." ("Boolean Text.Text")) -> (error out=w386:errorcluster)  [unwired: 1 in, 1 out]
        n125 = Unbundle(w418) -> ("Ctrl"=w416:refnum<vi>)  [unwired: 1 out]
        n126 = property class="Ctl"(reference=w416, error in=w417) -> ("Label.Text"=w413:string)  [unwired: 2 out]
        n127 = call "Enqueue Message.vi"("error in"=w386, "Message"="Graph.Update", "Queue"=w422) -> ("error out"=w411:errorcluster, "Queue dup."=w412:refnum<queue>)  [unwired: 7 in]
        n128 = case shown="\"Frequency\"" w413 {
          tunnel: w412 -> [_ w457 _]
          tunnel: w411 -> [w448 w454 w461]
          tunnel: [w448 w450 w459] -> w447
          frame Default {
          }
          frame "Frequency" {
            n129 = call "Enqueue Message.vi"("error in"=w454, "Message"="SyncParameters.Update", "Queue"=w457) -> ("error out"=w453:errorcluster, "Queue dup."=w458:refnum<queue>)  [unwired: 7 in]
            n130 = call "Enqueue Message.vi"("error in"=w453, "Message"="SyncParameters.Reset", "Queue"=w458) -> ("error out"=w451:errorcluster, "Queue dup."=w452:refnum<queue>)  [unwired: 7 in]
            n131 = call "Enqueue Message.vi"("error in"=w451, "Message"="Interaction.updateParameters", "Queue"=w452) -> ("error out"=w450:errorcluster)  [unwired: 7 in, 1 out]
          }
          frame "RaPF" {
            n132 = property on="RaPF" class="Bool (strict)"(error in=w461) -> (error out=w460:errorcluster, "Value"=w462:bool)  [unwired: 1 in, 1 out]
            n133 = Select(t=T10."Enabled" ("Disabled"), s=w462, f=T10."Disabled and Grayed Out" ("Disabled")) -> (s? t:f=w463:T10)
            n134 = property on="Cut Off" class="DigNum (strict)"(error in=w460, "DisabledEnum"=w463) -> (error out=w459:errorcluster)  [unwired: 1 in, 1 out]
          }
        }
        n135 = call "FGVCalibrations.vi"("Enum"=Enum."Read") -> ("calibOut"=w436:T20)  [unwired: 9 in, 1 out]
        n136 = Unbundle By Name(w436) -> ("calibParameters"=w437:T21, "calibIndex"=w434:i32)
        n137 = call "FGVfpgaAdress.vi"("Enum"=Enum."Read") -> ("voltageRange(+/-)Out"=w394:dbl, "ioFreqHzOut"=w405:u32)  [unwired: 5 in, 4 out]
        n138 = Index Array(array=w437, index=w434) -> (element=w433:T22)
        n139 = Unbundle By Name(w433) -> ("Range.Range Z"=w430:dbl)
        n140 = local read "Excitation"() -> (w403:T3)
        n141 = Unbundle By Name(w403) -> ("DC Offset"=w432:dbl, "Amplitude"=w431:dbl, "Frequency"=w404:dbl, "Cut Off"=w408:dbl, "RaPF"=w440:bool, "Shift"=w439:dbl)
        n142 = property on="Type" class="Ring (strict)"() -> ("Strings []"=w420:string[], "Value"=w419:u16)  [unwired: 2 in, 2 out]
        n143 = local read "Type"() -> (w399:u16)
        n144 = Index Array(array=w420, index=w419) -> (element=w438:string)
        n145 = Equal?(x=w399, y=w398) -> (x = y?=w397:bool)
        n146 = call "corerceFPGAClock.vi"("baseClock"=w405, "requestedFrequency"=w404) -> ("realFrequency"=w401:dbl)  [unwired: 7 in, 2 out]
        n147 = Divide(x=w439, y=w407) -> (x/y=w409:dbl)
        n148 = Divide(x=w408, y=w407) -> (x/y=w406:dbl)
        n149 = case shown="\"Piezo\", Default" w438 {
          tunnel: w432 -> [w470 w472]
          tunnel: w431 -> [w469 w471]
          tunnel: w430 -> [w468 _]
          tunnel: [w467 w472] -> w429
          tunnel: [w466 w471] -> w428
          frame "Piezo", Default {
            n150 = Divide(x=w470, y=w468) -> (x/y=w467:dbl)
            n151 = Divide(x=w469, y=w468) -> (x/y=w466:dbl)
          }
          frame "Photothermal" {
          }
        }
        n152 = Select(t=w393, s=w397, f=10.0 ("y")) -> (s? t:f=w396:dbl)
        n153 = local read "Signal"() -> (w441:u16)
        n154 = Divide(x=w394, y=w396) -> (x/y=w389:dbl)
        n155 = Equal?(x=w394, y=w393) -> (x = y?=w395:bool)
        n156 = Bundle By Name(cluster=w403, "Frequency"=w401) -> (w402:T3)
        n157 = Bundle By Name(cluster=T13 {"DC Offset"=0.4, "amplitude"=0.20000000000000004, "frequency"=10000.0, "Signal Type"=4, "cutoff"=0.2, "RaPF"=TRUE, "shift"=0.0} ("excitationParameters"), "DC Offset"=w429, "amplitude"=w428, "frequency"=w401, "cutoff"=w406, "RaPF"=w440, "shift"=w409, "Signal Type"=w441) -> (w442:T13)
        n158 = Select(t=10.0, s=w395, f=1.0 ("t")) -> (s? t:f=w390:dbl)
        n159 = Multiply(x=w389, y=w390) -> (x*y=w388:dbl)
        n160 = local write "Excitation"(w402) -> ()
        n161 = call "ExcitationParameters_v2.vi"("heartBeatSimParams"="heartBeatSimParams", "outputRange"=w388, "error in"=w447, "excitationParameters"=w442, "ioFreqHz"=w405, "FPGA VI Reference In"=w445) -> ("error out"=w385:errorcluster, "WaveSize"=w423:i32, "FPGA VI Reference Out"=w444:T16, "Excitation"=w425:dbl[])  [unwired: 2 in]
        n162 = Initialize Array(0.0 ("element"), w423) -> (w426:dbl[])
        n163 = Build Array(w425, w426) -> (w424:dbl[][])
        n164 = property on="Excitation enable?" class="Bool (strict)"(error in=w385, "BoolText.Text"="Enable" ("Boolean Text.Text")) -> (error out=w384:errorcluster)  [unwired: 1 in, 1 out]
      }
      frame "Excitation.setScannerLimits" {
        n165 = call "FGVCalibrations.vi"("Enum"=Enum."Read") -> ("calibOut"=w503:T20)  [unwired: 9 in, 1 out]
        n166 = Unbundle By Name(w503) -> ("calibParameters"=w504:T21, "calibIndex"=w501:i32)
        n167 = local read "Excitation"() -> (w487:T3)
        n168 = Index Array(array=w504, index=w501) -> (element=w500:T22)
        n169 = Unbundle By Name(w487) -> ("Amplitude"=w485:dbl, "DC Offset"=w486:dbl)
        n170 = property on="Type" class="Ring (strict)"() -> ("Strings []"=w484:string[], "Value"=w483:u16)  [unwired: 2 in, 2 out]
        n171 = Unbundle By Name(w500) -> ("Range.Range Z"=w497:dbl)
        n172 = Index Array(array=w484, index=w483) -> (element=w498:string)
        n173 = xnode "Read/Write Control"("FPGA VI Reference In"=w479, "error in"=w482) -> ("FPGA VI Reference Out"=w481:T16, "error out"=w480:errorcluster, "fb.p.limits"=w474:T9, "fb.loff.p.params"=w499:T23)
        n174 = case shown="\"Photothermal\"" w498 {
          tunnel: [T9 {"upperLimit"=1.0, "lowerLimit"=-1.0} ("fb.p.limits") w528] -> w489
          tunnel: w499 -> [w507 w527]
          tunnel: [w507 w526] -> w488
          tunnel: w497 -> [_ w523]
          tunnel: w474 -> [_ w525]
          tunnel: w486 -> [_ w518]
          tunnel: w485 -> [_ w517]
          frame "Photothermal" {
          }
          frame "ZPiezo", Default {
            w508 = 2.0 ("value")
            w522 = -1.0 ("lower limit")
            w524 = 1.0 ("upper limit")
            n175 = property on="Amplitude" class="DigNum (strict)"("Maximum"=w523) -> ()  [unwired: 2 in, 2 out]
            n176 = Add(x=w517, y=w518) -> (x+y=w519:dbl)
            n177 = Divide(x=w517, y=w523) -> (x/y=w511:dbl)
            n178 = Divide(x=w519, y=w523) -> (x/y=w509:dbl)
            n179 = Compound Arithmetic op=MULTIPLY(w509, w508) -> (w513:dbl)
            n180 = Compound Arithmetic op=MULTIPLY(w508, w511) -> (w512:dbl)
            n181 = Subtract(x=1.0, y=w513) -> (x-y=w514:dbl)
            n182 = Add(x=-1.0, y=w512) -> (x+y=w510:dbl)
            n183 = In Range and Coerce(upper limit=w524, x=w514, lower limit=w522) -> (coerced(x)=w521:dbl)  [unwired: 1 out]
            n184 = In Range and Coerce(upper limit=w524, x=w510, lower limit=w522) -> (coerced(x)=w520:dbl)  [unwired: 1 out]
            n185 = Bundle By Name(cluster=w525, "upperLimit"=w521, "lowerLimit"=w520) -> (w528:T9)
            n186 = Bundle By Name(cluster=w527, "disengagePos"=w520) -> (w526:T23)
          }
        }
        n187 = local read "Excitation"() -> (w477:T3)
        n188 = local read "Signal"() -> (w495:u16)
        n189 = call "FGVExcitationParameters.vi"("Enum"=Enum."Read") -> ("lineFitThreshold Out"=w492:dbl, "syncParameters Out"=w493:T24, "Sensitivities Out"=w490:T25, "Excitation Out"=w491:T14)  [unwired: 6 in, 1 out]
        n190 = Bundle By Name(cluster=w491, "Excitation"=w477, "Signal"=w495) -> (w476:T14)
        n191 = call "FGVExcitationParameters.vi"("Excitation In"=w476, "Enum"=Enum."Write", "lineFitThreshold In"=w492, "syncParameters In"=w493, "Sensitivities In"=w490) -> ()  [unwired: 2 in, 5 out]
        n192 = xnode "Read/Write Control"("FPGA VI Reference In"=w481, "error in"=w480, "fb.p.limits"=w489, "fb.loff.p.params"=w488) -> ("FPGA VI Reference Out"=w478:T16, "error out"=w473:errorcluster)
      }
      frame " -------- Background --------" {
      }
      frame "Background.Correct" {
        n193 = xnode "Invoke Method"("FPGA VI Reference In"=w534, "error in"=w536, "IRQ Number(s)"=4) -> ("FPGA VI Reference Out"=w533:T16, "error out"=w535:errorcluster)
        n194 = call "Enqueue Message.vi"("error in"=w535, "Message"="SyncParameters.Update", "Queue"=w544) -> ("error out"=w540:errorcluster, "Queue dup."=w545:refnum<queue>)  [unwired: 7 in]
        n195 = call "Enqueue Message.vi"("error in"=w540, "Message"="Background.WaitonIRQ4", "Queue"=w545) -> ("error out"=w539:errorcluster)  [unwired: 7 in, 1 out]
      }
      frame "Background.Substract" {
        w551 = TRUE ("hdt.int.p.startTransfer")
        w557 = u8 0 items=["memoryChan1", "memoryChan2", "processVarFixedNoPts", "processVarStream"] ("hdt.int.s.transferSource")
        w564 = u8 1 items=["memoryChan1", "memoryChan2", "processVarFixedNoPts", "processVarStream"] ("hdt.int.s.transferSource")
        w601 = 20.0  # threshold
        w611 = 4 ("IRQ Number(s)")
        # "20"
        # "Photothermal"
        n196 = xnode "Invoke Method"("FPGA VI Reference In"=w610, "error in"=w591, "IRQ Number(s)"=w611, "Timeout (ms)"=100) -> ("FPGA VI Reference Out"=w613:T16, "error out"=w614:errorcluster)  [unwired: 2 out]
        n197 = xnode "Invoke Method"("FPGA VI Reference In"=w613, "error in"=w614, "IRQ Number(s)"=w611) -> ("FPGA VI Reference Out"=w569:T16, "error out"=w568:errorcluster)
        n198 = xnode "Read/Write Control"("FPGA VI Reference In"=w569, "error in"=w568) -> ("FPGA VI Reference Out"=w566:T16, "error out"=w565:errorcluster, "hdt.int.p.readParams"=w567:T17)
        n199 = Bundle By Name(cluster=w567, "hdt.int.s.transferSource"=w564, "hdt.int.p.startTransfer"=w551) -> (w558:T17)
        n200 = call "FGVBackgroundORT.vi"("Enum"=Enum."Read") -> ("error out"=w552:errorcluster, "arrayOut"=w553:i16[], "Wave Out"=w554:dbl[], "Wave Out Shifted"=w547:dbl[])  [unwired: 6 in, 1 out]
        n201 = call "FGVBackgroundORT.vi"("Corrected...In"=w551, "Enum"=Enum."Write", "error in"=w552, "arrayIn"=w553, "Wave In"=w554, "Wave In Shifted"=w547) -> ()  [unwired: 1 in, 5 out]
        n202 = xnode "Read/Write Control"("FPGA VI Reference In"=w566, "error in"=w565, "hdt.int.p.readParams"=w558) -> ("FPGA VI Reference Out"=w571:T16, "error out"=w570:errorcluster)
        n203 = xnode "Invoke Method"("FPGA VI Reference In"=w571, "error in"=w570, "Number of Elements"=u32 0, "Timeout (ms)"=100) -> ("FPGA VI Reference Out"=w575:T16, "error out"=w574:errorcluster, "Elements Remaining"=w573:u32)  [unwired: 1 out]
        n204 = local read "Synchronization"() -> (w594:T2)
        n205 = local read "Sensitivities"() -> (w595:cluster{"Input":dbl, "Output":dbl})
        n206 = Unbundle By Name(w595) -> ("Input"=w592:dbl)
        n207 = xnode "Invoke Method"("FPGA VI Reference In"=w575, "error in"=w574, "Number of Elements"=w573, "Timeout (ms)"=100) -> ("FPGA VI Reference Out"=w563:T16, "error out"=w561:errorcluster, "Data"=w548:i16[])  [unwired: 1 out]
        n208 = Bundle By Name(cluster=w558, "hdt.int.s.transferSource"=w557) -> (w559:T17)
        n209 = Unbundle By Name(w594) -> ("Average Band"=w606:u16)
        n210 = Multiply(x=w592, y=w548) -> (x*y=w590:dbl[])
        n211 = Build Array (concatenate)(w590, w590) -> (w602:dbl[])
        n212 = Divide(x=w584, y=u32 4) -> (x/y=w600:dbl)
        n213 = Decrement(x=w606) -> (x-1=w607:u16)
        n214 = call <vilib>:"Peak Detector.vi"("peaks/valleys"=enum32{"Peaks", "Valleys"}."Valleys", "width"=w600, "threshold"=w601, "X"=w602) -> ("Locations"=w604:dbl[])  [unwired: 3 in, 4 out]
        n215 = Scale By Power Of 2(n=w607, x=ext 1.0) -> (x*2^n=w609:ext)
        n216 = Index Array(array=w604, index=0) -> (element=w605:dbl)
        n217 = xnode "Read/Write Control"("FPGA VI Reference In"=w563, "error in"=w561, "hdt.int.p.readParams"=w559, "ort.bgc.p.start"=TRUE) -> ("FPGA VI Reference Out"=w562:T16, "error out"=w560:errorcluster)
        n218 = Subtract(x=w605, y=w609) -> (x-y=w597:ext)
        n219 = Quotient & Remainder(x=w597, y=w584) -> (x-y*floor(x/y)=w580:ext)  [unwired: 1 out]
        n220 = Bundle By Name(cluster=w594, "syncPoint"=w580, "Use SyncPoint"=TRUE) -> (w596:T2)
        n221 = call "FGVBackgroundORT.vi"("Enum"=Enum."Read", "error in"=w560) -> ("error out"=w578:errorcluster, "Wave Out"=w588:dbl[], "Wave Out Shifted"=w546:dbl[])  [unwired: 5 in, 2 out]
        n222 = call "FGVBackgroundORT.vi"("Corrected...In"=FALSE, "Enum"=Enum."Write", "error in"=w578, "arrayIn"=w548, "Wave In"=w588, "Wave In Shifted"=w546) -> ("error out"=w579:errorcluster)  [unwired: 1 in, 4 out]
        n223 = local write "Synchronization"(w596) -> ()
        n224 = property on="Background" class="Bool (strict)"(error in=w579, "DisabledEnum"=T10."Enabled" ("Disabled")) -> (error out=w586:errorcluster)  [unwired: 1 in, 1 out]
        n225 = Replace Array Subset(array=w582, new element=w548, index (row)=1 ("disabled index (col)")) -> (w581:dbl[][])  [unwired: 1 in]
      }
      frame "Background.WaitonIRQ4" {
        w622 = 4 ("IRQ Number(s)")
        n226 = xnode "Invoke Method"("FPGA VI Reference In"=w621, "error in"=w615, "IRQ Number(s)"=w622, "Timeout (ms)"=100) -> ("FPGA VI Reference Out"=w624:T16, "error out"=w625:errorcluster, "Timed Out"=w617:bool)  [unwired: 1 out]
        n227 = case shown="False" w617 {
          tunnel: w625 -> [w679 w684]
          tunnel: w624 -> [w678 w687]
          tunnel: w622 -> [w677 _]
          tunnel: [w659 w687] -> w619
          tunnel: [w650 w682] -> w618
          tunnel: w626 -> [w681 w685]
          frame False {
            w673 = TRUE ("hdt.int.p.startTransfer")
            w664 = u8 0 items=["memoryChan1", "memoryChan2", "processVarFixedNoPts", "processVarStream"] ("hdt.int.s.transferSource")
            w668 = u8 1 items=["memoryChan1", "memoryChan2", "processVarFixedNoPts", "processVarStream"] ("hdt.int.s.transferSource")
            n228 = xnode "Invoke Method"("FPGA VI Reference In"=w678, "error in"=w679, "IRQ Number(s)"=w677) -> ("FPGA VI Reference Out"=w638:T16, "error out"=w660:errorcluster)
            n229 = xnode "Invoke Method"("FPGA VI Reference In"=w638, "Number of Elements"=u32 0, "Timeout (ms)"=20) -> ("FPGA VI Reference Out"=w639:T16, "Elements Remaining"=w642:u32)  [unwired: 1 in, 2 out]
            n230 = xnode "Invoke Method"("FPGA VI Reference In"=w639, "Number of Elements"=w642, "Timeout (ms)"=100) -> ("FPGA VI Reference Out"=w637:T16)  [unwired: 1 in, 3 out]
            n231 = xnode "Read/Write Control"("FPGA VI Reference In"=w637, "error in"=w660) -> ("FPGA VI Reference Out"=w670:T16, "error out"=w669:errorcluster, "hdt.int.p.readParams"=w671:T17)
            n232 = Bundle By Name(cluster=w671, "hdt.int.s.transferSource"=w668, "hdt.int.p.startTransfer"=w673) -> (w661:T17)
            n233 = call "FGVBackgroundORT.vi"("Enum"=Enum."Read") -> ("error out"=w676:errorcluster, "arrayOut"=w674:i16[], "Wave Out"=w675:dbl[], "Wave Out Shifted"=w627:dbl[])  [unwired: 6 in, 1 out]
            n234 = call "FGVBackgroundORT.vi"("Corrected...In"=w673, "Enum"=Enum."Write", "error in"=w676, "arrayIn"=w674, "Wave In"=w675, "Wave In Shifted"=w627) -> ()  [unwired: 1 in, 5 out]
            n235 = xnode "Read/Write Control"("FPGA VI Reference In"=w670, "error in"=w669, "hdt.int.p.readParams"=w661) -> ("FPGA VI Reference Out"=w634:T16, "error out"=w635:errorcluster, "ort.p.waveSize"=w636:u16)
            n236 = xnode "Invoke Method"("FPGA VI Reference In"=w634, "error in"=w635, "Number of Elements"=w636, "Timeout (ms)"=100) -> ("FPGA VI Reference Out"=w667:T16, "error out"=w666:errorcluster, "Data"=w645:i16[])  [unwired: 1 out]
            n237 = Bundle By Name(cluster=w661, "hdt.int.s.transferSource"=w664) -> (w665:T17)
            n238 = property on="Type" class="Ring (strict)"() -> ("Strings []"=w654:string[], "Value"=w653:u16)  [unwired: 2 in, 2 out]
            n239 = Index Array(array=w654, index=w653) -> (element=w657:string)
            n240 = xnode "Read/Write Control"("FPGA VI Reference In"=w667, "error in"=w666, "hdt.int.p.readParams"=w665) -> ("FPGA VI Reference Out"=w659:T16, "error out"=w652:errorcluster)
            n241 = Equal?(x=w657, y="ZPiezo") -> (x = y?=w658:bool)
            n242 = call "FGVBackgroundORT.vi"("Enum"=Enum."Read") -> ("error out"=w648:errorcluster, "Wave Out"=w647:dbl[], "Wave Out Shifted"=w628:dbl[])  [unwired: 6 in, 2 out]
            n243 = Select(t="Background.ZPiezo" ("Message"), s=w658, f="Background.Photothermal" ("Message")) -> (s? t:f=w655:string)
            n244 = call "FGVBackgroundORT.vi"("Corrected...In"=FALSE, "Enum"=Enum."Write", "error in"=w648, "arrayIn"=w645, "Wave In"=w647, "Wave In Shifted"=w628) -> ()  [unwired: 1 in, 5 out]
            n245 = call "Enqueue Message.vi"("error in"=w652, "Message"=w655, "Queue"=w681) -> ("error out"=w631:errorcluster, "Queue dup."=w680:refnum<queue>)  [unwired: 7 in]
            n246 = property on="Background" class="Bool (strict)"(error in=w631, "Value"=FALSE ("Background")) -> (error out=w630:errorcluster)  [unwired: 1 in, 1 out]
            n247 = call "Enqueue Message.vi"("error in"=w630, "Message"="Graph.Update", "Queue"=w680) -> ("error out"=w650:errorcluster)  [unwired: 7 in, 1 out]
          }
          frame True {
            n248 = Wait (ms)(milliseconds to wait=u32 50) -> ()  [unwired: 1 out]
            n249 = call "Enqueue Message.vi"("error in"=w684, "Message"="Background.WaitonIRQ4", "Queue"=w685) -> ("error out"=w682:errorcluster)  [unwired: 7 in, 1 out]
          }
        }
      }
      frame "Background.Photothermal" {
        w709 = 20.0  # threshold
        # "Photothermal"
        n250 = call "FGVBackgroundORT.vi"("Enum"=Enum."Read", "error in"=w689) -> ("error out"=w718:errorcluster, "arrayOut"=w690:i16[])  [unwired: 5 in, 3 out]
        n251 = local read "Sensitivities"() -> (w703:cluster{"Input":dbl, "Output":dbl})
        n252 = Unbundle By Name(w703) -> ("Input"=w701:dbl)
        n253 = local read "Synchronization"() -> (w702:T2)
        n254 = Multiply(x=w701, y=w690) -> (x*y=w700:dbl[])
        n255 = Build Array (concatenate)(w700, w700) -> (w710:dbl[])
        n256 = Divide(x=w696, y=u32 4) -> (x/y=w708:dbl)
        n257 = Unbundle By Name(w702) -> ("Average Band"=w714:u16)
        n258 = call <vilib>:"Peak Detector.vi"("peaks/valleys"=enum32{"Peaks", "Valleys"}."Valleys", "width"=w708, "threshold"=w709, "X"=w710) -> ("Locations"=w712:dbl[])  [unwired: 3 in, 4 out]
        n259 = Decrement(x=w714) -> (x-1=w715:u16)
        n260 = Index Array(array=w712, index=0) -> (element=w713:dbl)
        n261 = Scale By Power Of 2(n=w715, x=ext 1.0) -> (x*2^n=w717:ext)
        n262 = Subtract(x=w713, y=w717) -> (x-y=w705:ext)
        n263 = Quotient & Remainder(x=w705, y=w696) -> (x-y*floor(x/y)=w692:ext)  [unwired: 1 out]
        n264 = Bundle By Name(cluster=w702, "syncPoint"=w692, "Use SyncPoint"=TRUE) -> (w704:T2)
        n265 = local write "Synchronization"(w704) -> ()
        n266 = property on="Background" class="Bool (strict)"(error in=w718, "DisabledEnum"=T10."Enabled" ("Disabled")) -> (error out=w698:errorcluster)  [unwired: 1 in, 1 out]
        n267 = Replace Array Subset(array=w694, new element=w690, index (row)=1 ("disabled index (col)")) -> (w693:dbl[][])  [unwired: 1 in]
      }
      frame "Background.Frame" {
        n268 = Variant To Data(error in=w731, type=refnum<vi> refnum ("CtlRef"), Variant=w730) -> (data=w728:refnum<vi>, error out=w727:errorcluster)
        n269 = property class="Ctl"(reference=w728, error in=w727) -> (reference out=w725:refnum<vi>, error out=w724:errorcluster, "Label.Text"=w726:string)
        n270 = case shown="\"Request\"" w726 {
          tunnel: w725 -> [w741 w752]
          tunnel: w724 -> [w740 w753]
          tunnel: w723 -> [w734 w745]
          tunnel: [w733 w745] -> w722
          tunnel: [w732 w748] -> w721
          frame "Correction", Default {
            n271 = To More Specific Class(target class=refnum<vi> refnum ("Correction"), reference=w741, error in=w740) -> (specific class reference=w738:refnum<vi>, error out=w737:errorcluster)
            n272 = property class="Bool (strict)"(reference=w738, error in=w737) -> (error out=w736:errorcluster, "Value"=w735:bool)  [unwired: 1 out]
            n273 = xnode "Read/Write Control"("FPGA VI Reference In"=w734, "error in"=w736, "itc.p.allowBGC"=w735) -> ("FPGA VI Reference Out"=w733:T16, "error out"=w732:errorcluster)
          }
          frame "Request" {
            n274 = To More Specific Class(target class=refnum<vi> refnum ("Request"), reference=w752, error in=w753) -> (specific class reference=w751:refnum<vi>, error out=w750:errorcluster)
            n275 = property class="Enum (strict)"(reference=w751, error in=w750) -> (error out=w744:errorcluster, "Value"=w749:enum16{"Never", "End of line", "End of frame"})  [unwired: 1 out]
            n276 = call "FGVfpgaAdressScanEngine.vi"("Enum"=Enum."Read", "error in"=w744) -> ("error out"=w743:errorcluster, "FPGA.SEout"=w742:T19)  [unwired: 5 in, 3 out]
            n277 = xnode "Read/Write Control"("FPGA VI Reference In"=w742, "error in"=w743, "ort.bgc.requestType"=w749) -> ("error out"=w748:errorcluster)  [unwired: 1 out]
          }
        }
      }
      frame " ----- Synchronization ----- " {
      }
      frame "SyncParameters.Update" {
        w800 = T26 {"intOutMAEnable"=FALSE, "bgcAverageCount"=0, "waveSize"=0, "resetBGC"=FALSE, "liftHeight"=0.0}  # BackgroundParameters
        n278 = local read "Synchronization"() -> (w789:T2)
        n279 = call "FGVCalibrations.vi"("Enum"=Enum."Read") -> ("calibOut"=w783:T20)  [unwired: 9 in, 1 out]
        n280 = Unbundle By Name(w783) -> ("calibParameters"=w784:T21, "calibIndex"=w781:i32)
        n281 = Bundle By Name(cluster=w789, "Upper"=w775, "Lower"=u16 0 ("maxSearchLower")) -> (w774:T2)
        n282 = local read "Background-"() -> (w804:cluster{"Lift Height":dbl, "Average Count":u16})
        n283 = Unbundle By Name(w774) -> ("syncPoint"=w773:u16)
        n284 = Index Array(array=w784, index=w781) -> (element=w780:T22)
        n285 = call "FGVSyncPoint.vi"("Enum"=Enum."Write", "SyncPointIn"=w773) -> ("SyncPointOut"=w762:u16)  [unwired: 8 in, 1 out]
        n286 = Unbundle By Name(w804) -> ("Average Count"=w801:u16, "Lift Height"=w778:dbl)
        n287 = Unbundle By Name(w780) -> ("Range.Range Z"=w776:dbl)
        n288 = call "FGVBackgroundORT.vi"("Enum"=Enum."Read") -> ("error out"=w765:errorcluster, "arrayOut"=w766:i16[], "Wave Out"=w758:dbl[], "Corrected...Out"=w760:bool)  [unwired: 6 in, 1 out]
        n289 = Divide(x=w778, y=w776) -> (x/y=w779:dbl)
        n290 = Array Size(array=w758) -> (size(s)=w770:i32)
        n291 = Multiply(x=w779, y=2.0) -> (x*y=w777:dbl)
        n292 = Divide(x=w770, y=2 ("x")) -> (x/y=w768:dbl)
        n293 = Subtract(x=w762, y=w768) -> (x-y=w767:dbl)
        n294 = Rotate 1D Array(1:w758, 2:w767) -> (0:w759:dbl[])
        n295 = Bundle By Name(cluster=w800, "intOutMAEnable"="intOutMAEnable", "resetBGC"="Background", "bgcAverageCount"=w801, "liftHeight"=w777) -> (w798:T26)
        n296 = call "FGVBackgroundORT.vi"("Corrected...In"=w760, "Enum"=Enum."Write", "error in"=w765, "arrayIn"=w766, "Wave In"=w758, "Wave In Shifted"=w759) -> ()  [unwired: 1 in, 5 out]
        n297 = local read "Sensitivities"() -> (w792:cluster{"Input":dbl, "Output":dbl})
        n298 = local read "lineFitThreshold"() -> (w786:dbl)
        n299 = local read "Excitation"() -> (w761:T3)
        n300 = Unbundle By Name(w792) -> ("Input"=w791:dbl)
        n301 = call "SyncParameters.vi"("Excitation"=w761, "lineFitThreshold"=w786, "inputSensitivity"=w791, "error in"=w805, "syncParameters"=w774, "BackgroundParameters"=w798, "FPGA VI Reference In"=w806) -> ("error out"=w771:errorcluster, "FPGA VI Reference Out"=w802:T16)  [unwired: 3 in]
        n302 = local write "Synchronization"(w774) -> ()
        n303 = call "FGVExcitationParameters.vi"("Enum"=Enum."Read", "error in"=w771) -> ("error out"=w803:errorcluster, "Sensitivities Out"=w793:T25)  [unwired: 5 in, 3 out]
        n304 = Bundle By Name(cluster=w793, "inputSensitivity"=w791) -> (w796:T25)
        n305 = call "FGVExcitationParameters.vi"("Enum"=Enum."Write", "error in"=w803, "lineFitThreshold In"=w786, "syncParameters In"=w774, "Sensitivities In"=w796) -> ("error out"=w790:errorcluster)  [unwired: 2 in, 4 out]
      }
      frame "SyncParameters.Reset" {
        n306 = Multiply(x=w811, y=0.5) -> (x*y=w812:dbl)
        n307 = To Unsigned Word Integer(number=w812) -> (unsigned 16bit integer=w809:u16)
        n308 = property on="syncPoint" class="DigNum (strict)"("Val(Sgnl)"=w809) -> ()  [unwired: 2 in, 2 out]
        n309 = call "FGVSyncPoint.vi"("Enum"=Enum."Write", "error in"=w808, "SyncPointIn"=w809) -> ("error out"=w807:errorcluster)  [unwired: 7 in, 1 out]
      }
      frame "SyncParameters.Calculate" {
        w839 = TRUE ("hdt.int.p.startTransfer")
        w848 = u8 0 items=["memoryChan1", "memoryChan2", "processVarFixedNoPts", "processVarStream"] ("hdt.int.s.transferSource")
        w854 = u8 1 items=["memoryChan1", "memoryChan2", "processVarFixedNoPts", "processVarStream"] ("hdt.int.s.transferSource")
        w849 = 1 ("disabled index (col)")
        # "Removed UseSynchPoint to true"
        # "ZPiezo Excitation"
        n310 = xnode "Read/Write Control"("FPGA VI Reference In"=w834, "error in"=w835) -> ("FPGA VI Reference Out"=w855:T16, "error out"=w826:errorcluster, "hdt.int.p.readParams"=w837:T17)
        n311 = Bundle By Name(cluster=w837, "hdt.int.s.transferSource"=w854) -> (w836:T17)
        n312 = Bundle By Name(cluster=w836, "hdt.int.p.startTransfer"=w839) -> (w838:T17)
        n313 = xnode "Read/Write Control"("FPGA VI Reference In"=w855, "error in"=w826, "hdt.int.p.readParams"=w836, "hdt.int.p.readParams"=w838) -> ("FPGA VI Reference Out"=w833:T16, "error out"=w828:errorcluster)
        n314 = call "FGVBackgroundORT.vi"("Enum"=Enum."Read", "error in"=w826) -> ("error out"=w840:errorcluster, "arrayOut"=w841:i16[], "Wave Out"=w842:dbl[], "Wave Out Shifted"=w821:dbl[])  [unwired: 5 in, 1 out]
        n315 = call "FGVBackgroundORT.vi"("Corrected...In"=w839, "Enum"=Enum."Write", "error in"=w840, "arrayIn"=w841, "Wave In"=w842, "Wave In Shifted"=w821) -> ()  [unwired: 1 in, 5 out]
        n316 = xnode "Invoke Method"("FPGA VI Reference In"=w833, "error in"=w828, "IRQ Number(s)"=4 ("Background"), "Timeout (ms)"=-1) -> ("FPGA VI Reference Out"=w832:T16, "error out"=w829:errorcluster, "IRQ(s) Asserted"=w827:i32)  [unwired: 1 out]
        n317 = xnode "Invoke Method"("FPGA VI Reference In"=w832, "error in"=w829, "IRQ Number(s)"=w827) -> ("FPGA VI Reference Out"=w831:T16, "error out"=w830:errorcluster)
        n318 = xnode "Invoke Method"("FPGA VI Reference In"=w831, "error in"=w830, "Number of Elements"=u32 0, "Timeout (ms)"=400) -> ("FPGA VI Reference Out"=w859:T16, "error out"=w858:errorcluster, "Elements Remaining"=w857:u32)  [unwired: 1 out]
        n319 = Bundle By Name(cluster=w836, "hdt.int.s.transferSource"=w848) -> (w847:T17)
        n320 = xnode "Invoke Method"("FPGA VI Reference In"=w859, "error in"=w858, "Number of Elements"=w857, "Timeout (ms)"=20) -> ("FPGA VI Reference Out"=w853:T16, "error out"=w852:errorcluster, "Data"=w824:i16[])  [unwired: 1 out]
        n321 = local read "Sensitivities"() -> (w870:cluster{"Input":dbl, "Output":dbl})
        n322 = xnode "Read/Write Control"("FPGA VI Reference In"=w853, "error in"=w852, "hdt.int.p.readParams"=w847) -> ("FPGA VI Reference Out"=w850:T16, "error out"=w851:errorcluster)
        n323 = call "FGVBackgroundORT.vi"("Enum"=Enum."Read") -> ("error out"=w817:errorcluster, "Wave Out"=w818:dbl[], "Wave Out Shifted"=w819:dbl[])  [unwired: 6 in, 2 out]
        n324 = Unbundle By Name(w870) -> ()  [unwired: 1 out]
        n325 = call "FGVBackgroundORT.vi"("Corrected...In"=FALSE, "Enum"=Enum."Write", "error in"=w817, "arrayIn"=w824, "Wave In"=w818, "Wave In Shifted"=w819) -> ("arrayOut"=w823:i16[])  [unwired: 1 in, 4 out]
        n326 = xnode "Read/Write Control"("FPGA VI Reference In"=w850, "error in"=w851) -> ("FPGA VI Reference Out"=w866:T16, "error out"=w872:errorcluster, "ort.p.methodParams.ort.p.syncPoint"=w865:u16)
        n327 = Multiply(x=w823, y=1.0) -> (x*y=w863:dbl[])
        n328 = local read "Synchronization"() -> (w871:T2)
        n329 = Bundle By Name(cluster=w871, "syncPoint"=w865) -> (w869:T2)
        n330 = Delete From Array(array=w846, length=w845, index (row)=w849) -> (array with subset deleted=w864:dbl[][])  [unwired: 1 in, 1 out]
        n331 = local write "Synchronization"(w869) -> ()
        n332 = Insert Into Array(array=w864, index (row)=w849, new element=w863) -> (w862:dbl[][])  [unwired: 1 in]
      }
      frame "Background.ZPiezo" {
        w881 = 1 ("disabled index (col)")
        # "ZPiezo Excitation"
        n333 = call "FGVBackgroundORT.vi"("Enum"=Enum."Read", "error in"=w877) -> ("error out"=w887:errorcluster, "arrayOut"=w873:i16[])  [unwired: 5 in, 3 out]
        n334 = xnode "Read/Write Control"("FPGA VI Reference In"=w878, "error in"=w887) -> ("FPGA VI Reference Out"=w884:T16, "error out"=w886:errorcluster, "ort.p.methodParams.ort.p.syncPoint"=w874:u16)
        n335 = local read "Synchronization"() -> (w876:T2)
        n336 = Bundle By Name(cluster=w876, "syncPoint"=w874) -> (w875:T2)
        n337 = local write "Synchronization"(w875) -> ()
        n338 = Delete From Array(array=w880, length=w879, index (row)=w881) -> (array with subset deleted=w883:dbl[][])  [unwired: 1 in, 1 out]
        n339 = Insert Into Array(array=w883, index (row)=w881, new element=w873) -> (w882:dbl[][])  [unwired: 1 in]
      }
      frame " ----------- Graph ----------- " {
      }
      frame "Graph.Update" {
        # "0: Excitation\n1: Background"
        n340 = local read "Display"() -> (w897:u16)
        n341 = Transpose 2D Array(2D array=w899) -> (transposed array=w898:dbl[][])
        n342 = Index Array(array=w898, index (col)=w897) -> (element=w894:dbl[])  [unwired: 1 in]
        n343 = Array Size(array=w894) -> (size(s)=w893:i32)
        n344 = property on="Graph" class="WFGraph (strict)"(error in=w896, "XScale.Maximum"=w893, "XScale.Minimum"=0.0 ("X Scale.Range:Minimum")) -> (error out=w895:errorcluster)  [unwired: 1 in, 1 out]
        n345 = local write "Graph"(w894) -> ()
      }
      frame "------- Interaction Curve Display -------" {
      }
      frame "Interaction.updateParameters" {
        # "Number of ticks the FPGA waits before sending the next value from memory to the buffer. Should be >10."
        n346 = xnode "Read/Write Control"("FPGA VI Reference In"=w908, "error in"=w917) -> ("FPGA VI Reference Out"=w915:T16, "error out"=w910:errorcluster, "hdt.int.p.readParams"=w913:T17)
        n347 = Bundle By Name(cluster=w913, "hdt.int.p.memReadDec"=u16 20, "hdt.int.p.readLength"=w911) -> (w914:T17)
        n348 = xnode "Read/Write Control"("FPGA VI Reference In"=w915, "error in"=w910, "hdt.int.p.readParams"=w914) -> ("FPGA VI Reference Out"=w907:T16, "error out"=w909:errorcluster, "ort.p.methodParams.ort.p.useSyncPoint"=w916:bool)
        n349 = property on="Use SyncPoint" class="Bool (strict)"("Val(Sgnl)"=w916) -> ()  [unwired: 2 in, 2 out]
      }
      frame "--------- UserEvents ---------" {
      }
      frame "Menu.ChangeClock" {
        n350 = control-ref of="Frequency"() -> (w922:refnum<vi>)
        n351 = call "Enqueue Message.vi"("error in"=w924, "Data"=w922, "Message"="ExcitationParameters.Change", "Queue"=w929) -> ("error out"=w923:errorcluster)  [unwired: 6 in, 1 out]
      }
      frame "CursorMax.Move" {
        # "User Event: Reference Graph=> Cursor move"
        n352 = Variant To Data(error in=w949, type=0.0 ("X"), Variant=w948) -> (data=w941:dbl, error out=w950:errorcluster)
        n353 = call "FGVBackgroundORT.vi"("Enum"=Enum."Read") -> ("error out"=w935:errorcluster, "arrayOut"=w936:i16[], "Wave Out"=w931:dbl[])  [unwired: 6 in, 2 out]
        n354 = Array Size(array=w931) -> (size(s)=w940:i32)
        n355 = call "FGVSyncPoint.vi"("Enum"=Enum."Write", "error in"=w950, "SyncPointIn"=w941) -> ("error out"=w951:errorcluster, "SyncPointOut"=w930:u16)  [unwired: 7 in]
        n356 = Divide(x=w940, y=2 ("x")) -> (x/y=w938:dbl)
        n357 = Subtract(x=w930, y=w938) -> (x-y=w937:dbl)
        n358 = property on="syncPoint" class="DigNum (strict)"(error in=w951, "Value"=w930) -> (error out=w946:errorcluster)  [unwired: 1 in, 1 out]
        n359 = Rotate 1D Array(1:w931, 2:w937) -> (0:w932:dbl[])
        n360 = call "FGVBackgroundORT.vi"("Enum"=Enum."Write", "error in"=w935, "arrayIn"=w936, "Wave In"=w931, "Wave In Shifted"=w932) -> ()  [unwired: 2 in, 5 out]
      }
      frame "CursorMax.Release" {
        # "Update the SyncPoint Value when the cursor of the graph interaction curve is released"
        n361 = Variant To Data(error in=w976, type=0.0 ("X"), Variant=w975) -> (data=w963:dbl, error out=w971:errorcluster)
        n362 = xnode "Read/Write Control"("FPGA VI Reference In"=w970, "error in"=w971) -> ("FPGA VI Reference Out"=w969:T16, "error out"=w972:errorcluster, "ort.p.methodParams"=w973:T18)
        n363 = Bundle By Name(cluster=w973, "ort.p.syncPoint"=w963) -> (w974:T18)
        n364 = call "FGVBackgroundORT.vi"("Enum"=Enum."Read") -> ("error out"=w957:errorcluster, "arrayOut"=w958:i16[], "Wave Out"=w953:dbl[])  [unwired: 6 in, 2 out]
        n365 = xnode "Read/Write Control"("FPGA VI Reference In"=w969, "error in"=w972, "ort.p.methodParams"=w974) -> ("FPGA VI Reference Out"=w968:T16, "error out"=w967:errorcluster)
        n366 = Array Size(array=w953) -> (size(s)=w962:i32)
        n367 = call "FGVSyncPoint.vi"("Enum"=Enum."Write", "SyncPointIn"=w963) -> ("SyncPointOut"=w952:u16)  [unwired: 8 in, 1 out]
        n368 = Divide(x=w962, y=2 ("x")) -> (x/y=w960:dbl)
        n369 = Subtract(x=w952, y=w960) -> (x-y=w959:dbl)
        n370 = Rotate 1D Array(1:w953, 2:w959) -> (0:w954:dbl[])
        n371 = call "FGVBackgroundORT.vi"("Enum"=Enum."Write", "error in"=w957, "arrayIn"=w958, "Wave In"=w953, "Wave In Shifted"=w954) -> ()  [unwired: 2 in, 5 out]
      }
      frame "---Copy This Frame---" {
        n372 = Merge Errors(w982) -> (w981:errorcluster)
      }
      frame Default {
        n373 = Format Into String(format string="The message\"%s\" received in the gestion loop is not valid" ("Texte de message d'erreur inconnu"), w989) -> (resulting string=w986:string)  [unwired: 2 in, 1 out]
        n374 = call <vilib>:"Error Cluster From Error Code.vi"("error message (\"\")"=w986, "error code (0)"=1 ("code d'erreur (0)")) -> ("error out"=w987:errorcluster)  [unwired: 7 in]
      }
      frame "Initialize.FGV" {
        n375 = Bundle By Name(cluster=T14 {"Excitation"={"Frequency"=0.0, "Amplitude"=0.0, "DC Offset"=0.0, "Cut Off"=0.0, "RaPF"=FALSE, "Shift"=0.0}, "Background"={"Lift Height"=0.0, "Average Count"=12}, "Signal"=0} ("Excitation In"), "Excitation"="Excitation", "Background"="Background-") -> (w991:T14)
        n376 = call "FGVExcitationParameters.vi"("Excitation In"=w991, "Enum"=Enum."Write", "error in"=w1007, "lineFitThreshold In"="lineFitThreshold", "syncParameters In"="Synchronization", "Sensitivities In"="Sensitivities") -> ("error out"=w1008:errorcluster)  [unwired: 1 in, 4 out]
        n377 = Unbundle By Name("Excitation") -> ("DC Offset"=w1000:dbl, "Amplitude"=w999:dbl, "Frequency"=w998:dbl, "Cut Off"=w997:dbl, "RaPF"=w996:bool)
        n378 = Bundle By Name(cluster=T15 {"DC Offset"=0.0, "amplitude"=0.0, "frequency"=0.0, "Signal Type"=0, "cutoff"=0.0, "RaPF"=FALSE} ("excitationParameters"), "DC Offset"=w1000, "amplitude"=w999, "frequency"=w998, "cutoff"=w997, "RaPF"=w996, "Signal Type"="Signal") -> ()  [unwired: 1 out]
      }
    }
  }
  n379 = while {
    tunnel: w22 -> [w1018]
    tunnel: [w1014] -> w23
    tunnel: w17 -> [w1013]
    tunnel: [w1012] -> w16
    stop <- w1016 stop-if-true
    n380 = event shown="[4] \"Background\": Value Change" {
      selector: w1013 -> [_ _ _ _ _ _ _ _ _ _ _ _]
      dyn-events: [_ _ _ _ _ _ _ _ _ _ _ _] -> w1012
      timeout: 1 -> [_ _ _ _ _ _ _ _ _ _ _ _]
      tunnel: [w1033 _ _ _ _ _ _ _ _ _ _ TRUE ("Rejeter ?")] -> w1017
      tunnel: w1018 -> [w1028 w1034 w1041 w1045 w1051 w1061 w1066 w1069 w1076 w1081 w1086 w1087]
      tunnel: [w1032 _ w1037 w1047 w1049 w1062 w1063 w1067 w1073 w1079 w1083 _] -> w1014
      tunnel: [w1031 w1034 w1036 w1046 w1050 w1060 w1065 w1068 w1074 w1080 w1084 w1087] -> w1015
      event Panel Close? {
        w1033 = TRUE ("Rejeter ?")
        n381 = event-data() -> ()  [unwired: 1 in, 1 out]
        n382 = call "Enqueue Message.vi"("Prioritary message"=TRUE, "Data"=FALSE, "Message"="Excitation.Enable", "Queue"=w1028) -> ("Queue dup."=w1027:refnum<queue>)  [unwired: 6 in, 1 out]
        n383 = event-data ("Event Filter Node")("Discard?"=w1033) -> ()  [unwired: 1 in, 1 out]
        n384 = call "Enqueue Message.vi"("Prioritary message"=TRUE ("Message prioritaire ? (F)"), "Message"="Exit", "Queue"=w1027) -> ("error out"=w1032:errorcluster, "Queue dup."=w1031:refnum<queue>)  [unwired: 7 in]
      }
      event Timeout {
        n385 = event-data() -> ()  [unwired: 1 in, 3 out]
      }
      event "Type": Value Change {
        n386 = event-data() -> ()  [unwired: 1 in, 1 out]
        n387 = call "Enqueue Message.vi"("Message"="ExpConfig.Update", "Queue"=w1041) -> ("error out"=w1038:errorcluster, "Queue dup."=w1042:refnum<queue>)  [unwired: 8 in]
        n388 = control-ref of="Frequency"() -> (w1035:refnum<vi>)
        n389 = call "Enqueue Message.vi"("error in"=w1038, "Data"=w1035, "Message"="ExcitationParameters.Change", "Queue"=w1042) -> ("error out"=w1037:errorcluster, "Queue dup."=w1036:refnum<queue>)  [unwired: 6 in]
      }
      event "Excitation enable?": Value Change {
        n390 = event-data() -> ("NewVal"=w1043:bool)  [unwired: 1 in]
        n391 = call "Enqueue Message.vi"("Data"=w1043, "Message"="Excitation.Enable", "Queue"=w1045) -> ("error out"=w1047:errorcluster, "Queue dup."=w1046:refnum<queue>)  [unwired: 7 in]
      }
      event "Background": Value Change {
        n392 = event-data() -> ("NewVal"=w1048:bool)  [unwired: 1 in]
        n393 = case shown="True" w1048 {
          tunnel: w1051 -> [w1053 w1057]
          tunnel: [w1053 w1055] -> w1050
          tunnel: [errorcluster {"status"=FALSE, "code"=0, "source"=""} ("sortie d'erreur") w1054] -> w1049
          frame False {
          }
          frame True {
            n394 = call "Enqueue Message.vi"("Message"="Background.Correct", "Queue"=w1057) -> ("error out"=w1054:errorcluster, "Queue dup."=w1055:refnum<queue>)  [unwired: 8 in]
          }
        }
      }
      event "Excitation.Frequency", "Sensitivities.Output", "Signal", "Excitation.Amplitude", "Excitation.DC Offset", "Excitation.Cut Off", "Excitation.RaPF", "Excitation.Shift", "heartBeatSimParams": Value Change {
        n395 = event-data() -> ("CtlRef"=w1058:refnum<vi>)  [unwired: 1 in]
        n396 = call "Enqueue Message.vi"("Data"=w1058, "Message"="ExcitationParameters.Change", "Queue"=w1061) -> ("error out"=w1062:errorcluster, "Queue dup."=w1060:refnum<queue>)  [unwired: 7 in]
      }
      event "Synchronization", "intOutMAEnable", "lineFitThreshold", "Sensitivities.Input", "Background-": Value Change {
        n397 = event-data() -> ()  [unwired: 1 in, 4 out]
        n398 = call "Enqueue Message.vi"("Message"="SyncParameters.Update", "Queue"=w1066) -> ("error out"=w1063:errorcluster, "Queue dup."=w1065:refnum<queue>)  [unwired: 8 in]
      }
      event "Display": Value Change {
        n399 = event-data() -> ("NewVal"=w1071:u16)  [unwired: 1 in]
        n400 = call "Enqueue Message.vi"("Data"=w1071, "Message"="Graph.Update", "Queue"=w1069) -> ("error out"=w1067:errorcluster, "Queue dup."=w1068:refnum<queue>)  [unwired: 7 in]
      }
      event "Correction", "Request": Value Change {
        n401 = event-data() -> ("CtlRef"=w1072:refnum<vi>)  [unwired: 1 in]
        n402 = call "Enqueue Message.vi"("Data"=w1072, "Message"="Background.Frame", "Queue"=w1076) -> ("error out"=w1073:errorcluster, "Queue dup."=w1074:refnum<queue>)  [unwired: 7 in]
      }
      event Cursor Move {
        n403 = event-data() -> ("CursLoc.X"=w1077:dbl)  [unwired: 1 in]
        n404 = call "Enqueue Message.vi"("Data"=w1077, "Message"="CursorMax.Move", "Queue"=w1081) -> ("error out"=w1079:errorcluster, "Queue dup."=w1080:refnum<queue>)  [unwired: 7 in]
      }
      event Cursor Release {
        n405 = event-data() -> ("CursLoc.X"=w1082:dbl)  [unwired: 1 in]
        n406 = call "Enqueue Message.vi"("Data"=w1082, "Message"="CursorMax.Release", "Queue"=w1086) -> ("error out"=w1083:errorcluster, "Queue dup."=w1084:refnum<queue>)  [unwired: 7 in]
      }
      event User Event {
        n407 = event-data() -> ()  [unwired: 1 in, 1 out]
      }
    }
    n408 = case shown="Error" w1014 {
      tunnel: [w1019 TRUE ("Rejeter ?")] -> w1016
      tunnel: w1017 -> [w1019 _]
      tunnel: w1015 -> [_ w1022]
      frame No Error {
      }
      frame Error {
        n409 = call "Enqueue Message.vi"("Prioritary message"=TRUE ("Message prioritaire ? (F)"), "Message"="Exit", "Queue"=w1022) -> ()  [unwired: 7 in, 2 out]
      }
    }
  }
  n410 = Unregister For Events(event registration refnum=w16, error in=w23) -> (error out=w4:errorcluster)
  n411 = Merge Errors(w4, w21) -> (w7:errorcluster)
  n412 = call <vilib>:"Simple Error Handler.vi"("error in (no error)"=w7) -> ("error out"=w6:errorcluster)  [unwired: 4 in, 4 out]
  n413 = call "FGVFileServer.vi"("Enum"=EnumFGVHDT."Pop", "error in"=w6, "New VI"=w5) -> ("error out"=w2:errorcluster)  [unwired: 7 in, 1 out]
  n414 = call "Destroy User Event - Stop.vi"("entrée d'erreur (pas d'erreur)"=w2, "Événement utilisateur - Arrêt"=w1) -> ()  [unwired: 9 in, 1 out]
